vi "luch 2 in 1.vi"() -> ()   [LabVIEW 2016]
panel:
  out "Time Stamp":T1
  in  "stop":T2
  out "VISA resource name out":string
  out "I: DZ2K1W":string
  out "DZ2K1W":bool
  out "I: BZ2K1W":string
  out "BZ2K1W":bool
  out "I: BZ1K1W":string
  out "BZ1K1W":bool
  out "I: DZ1K1W":string
  out "DZ1K1W":bool
  out "I: F0-ethernet 5":string
  in  "F0-ethernet 5":bool
  out "F0-e 5":bool
  in  "GF":bool
  in  "FI":bool
  in  "F-R VISAR 4":bool
  in  "F-R VISAR 3":bool
  out "I: BZ1K2W":string
  out "BZ1K2W":bool
  out "I: DZ1K2W":string
  out "DZ1K2W":bool
  out "I: F0-ethernet 4":string
  in  "F0-ethernet 4":bool
  out "F0-e 4":bool
  out "I: BZ2K2W":string
  out "I: DZ2K2W":string
  out "DZ2K2W":bool
  out "BZ2K2W":bool
  in  "BK3":bool
  in  "BK 2":bool
  in  "BK1":bool
  in  "Kamera Y":bool
  out "mod 02":string
  out "mod 01":string
  in  "Setup":bool
  in  "Values start":T3=5 items=["External rising edge"=1, "Single shot internal rising edge"=3, "Single shot"=5]
  in  "DZ2K1W":bool
  in  "BZ2K1W":bool
  in  "BZ1K1W":bool
  in  "DZ1K1W":bool
  out "I F0-ethernet 1":string
  in  "F0-ethernet 1":bool
  out "F0-e 3":bool
  out "I: GF":string
  out "GF":bool
  in  "Delay D (0 s)":ext=100.0
  in  "GF":bool
  out "I: FI":string
  out "FI":bool
  in  "Delay C (0 s)":ext=100.0
  in  "FI":bool
  in  "F-R VISAR1":bool
  in  "Delay A (0 s)":ext=100.0
  out "F-R VISAR 1":bool
  out "I: F-R VISAR 1":string
  out "F-R VISAR 2":bool
  out "I: F-R VISAR 2":string
  in  "F-R VISAR2":bool
  in  "Delay B (0 s)":ext=100.0
  out "I F0-ethernet 3":string
  in  "F0-ethernet 3":bool
  out "F0-e 1":bool
  out "I: PZS 2 DOP":string
  out "I: PZS 1 DOP":string
  in  "PZS 2 DOP":bool
  in  "PZS 1 DOP":bool
  out "PZS 2 DOP":bool
  out "PZS 1 DOP":bool
  in  "BZ1K2W":bool
  in  "DZ1K2W":bool
  in  "BZ2K2W":bool
  in  "DZ2K2W":bool
  out "I: BK3":string
  out "BK3":bool
  in  "Delay H (0 s)":ext=100.0
  in  "BK3":bool
  in  "Delay G (0 s)":ext=100.0
  in  "BK2":bool
  out "I: BK2":string
  out "BK2":bool
  in  "Delay F (0 s)":ext=100.0
  in  "BK1":bool
  out "I: BK1":string
  out "BK1":bool
  out "I F0-ethernet 2":string
  in  "Delay E (0 s)":ext=100.0
  in  "Kamera Y":bool
  out "I: Kamera Y":string
  out "Kamera Y":bool
  in  "F0-ethernet 2":bool
  out "F0-e 2":bool
  out "error out 2":errorcluster
  out "I 0_3":string
  in  "rele 0_6":bool
  out "modul 03":string
  out "0_3":bool
  out "error out":errorcluster
  # "W1"
  # "Current(A)"
  # "FO-ETHERNET ¹5"
  # "2 CHANAL DZ"
  # "1 CHANAL DZ"
  # "Current(A)"
  # "Current(A)"
  # "2 CHANAL BZ"
  # "1 CHANAL BZ"
  # "Current(A)"
  # "Current(A)"
  # "W2"
  # "Current(A)"
  # "FO-ETHERNET ¹4"
  # "1 CHANAL DZ"
  # "2 CHANAL DZ"
  # "Current(A)"
  # "Current(A)"
  # "1 CHANAL BZ"
  # "2 CHANAL BZ"
  # "Current(A)"
  # "Current(A)"
  # "Current(A)"
  # "FO-ETHERNET ¹1"
  # "VISAR ¹2"
  # "VISAR ¹1"
  # "Current(A)"
  # "Current(A)"
  # "Delay (100~1099ns)"
  # "Delay (100~1099ns)"
  # "FORM IMPULSE"
  # "DEEP FRONT"
  # "Current(A)"
  # "Current(A)"
  # "Delay (100~1099ns)"
  # "Delay (100~1099ns)"
  # "Current(A)"
  # "FO-ETHERNET ¹3"
  # "PZS ¹1"
  # "PZS ¹2"
  # "Current(A)"
  # "Current(A)"
  # "Current(A)"
  # "FO-ETHERNET ¹2"
  # "KAMERA Y"
  # "KAMERA B1"
  # "Current(A)"
  # "Current(A)"
  # "Delay (100~1099ns)"
  # "Delay (100~1099ns)"
  # "KAMERA B2"
  # "KAMERA B3"
  # "Current(A)"
  # "Current(A)"
  # "Delay (100~1099ns)"
  # "Delay (100~1099ns)"
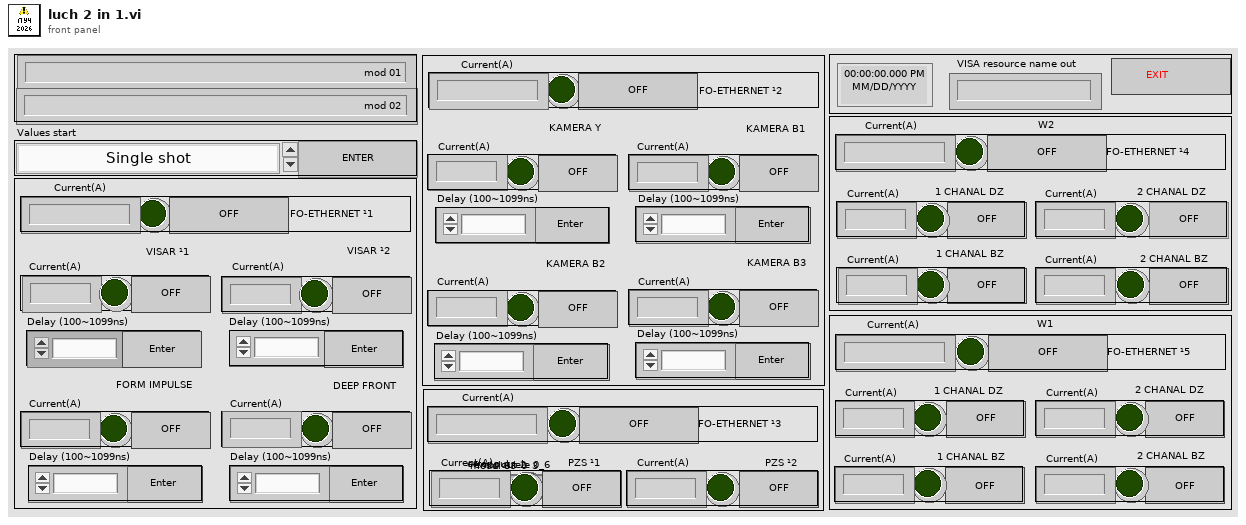
[diagram p1: front panel]
types:
  T1 = typedef "Control 4.ctl" = timestamp
  T2 = typedef "Control 1.ctl" = bool
  T3 = typedef "Control 2.ctl" = u16
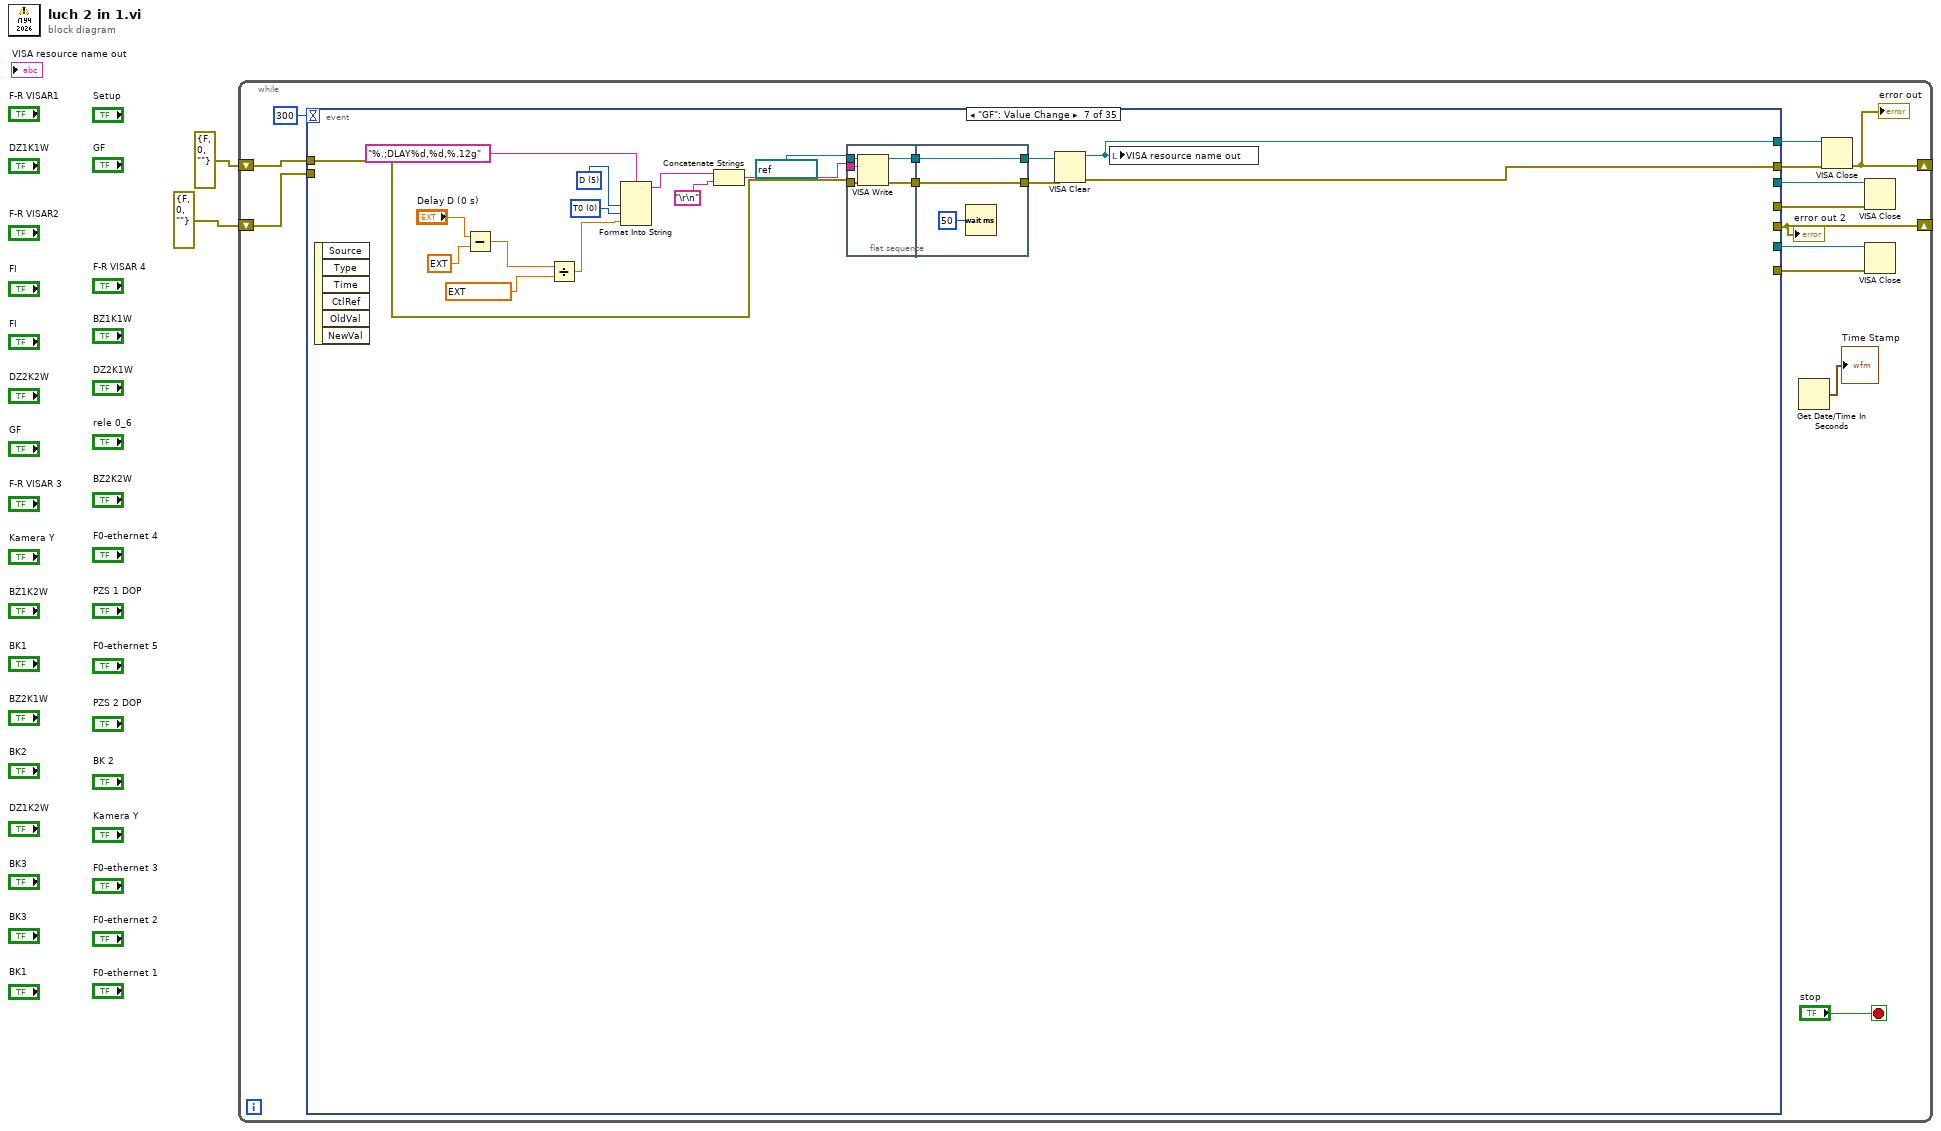
[diagram p0: block diagram]
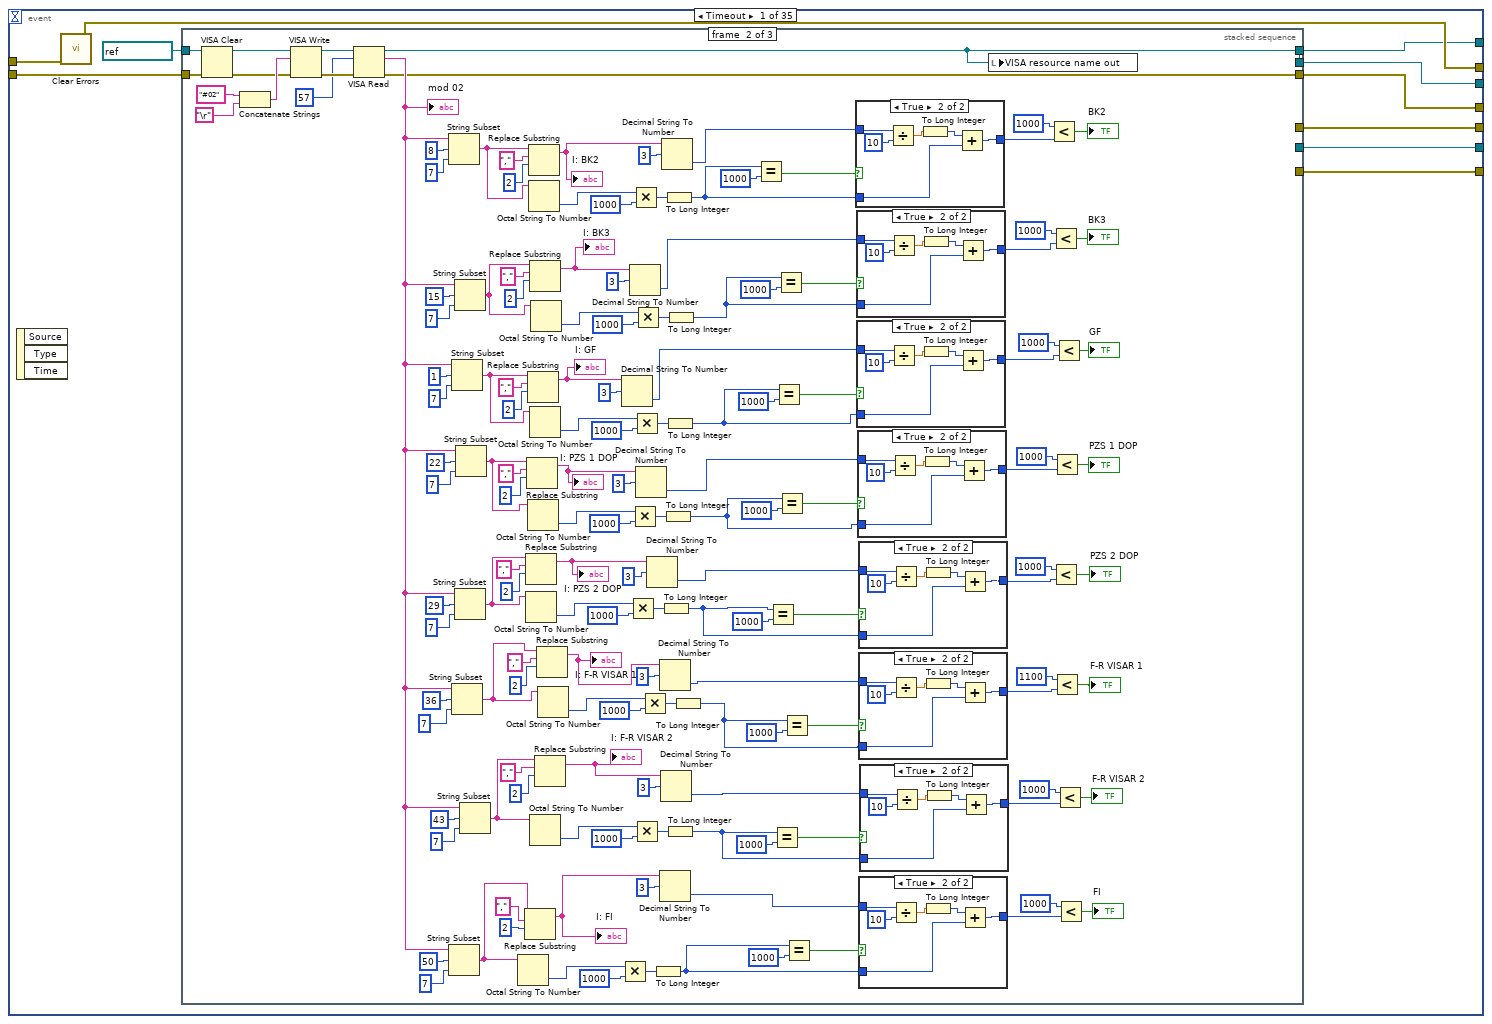
[diagram p2: hidden frame]
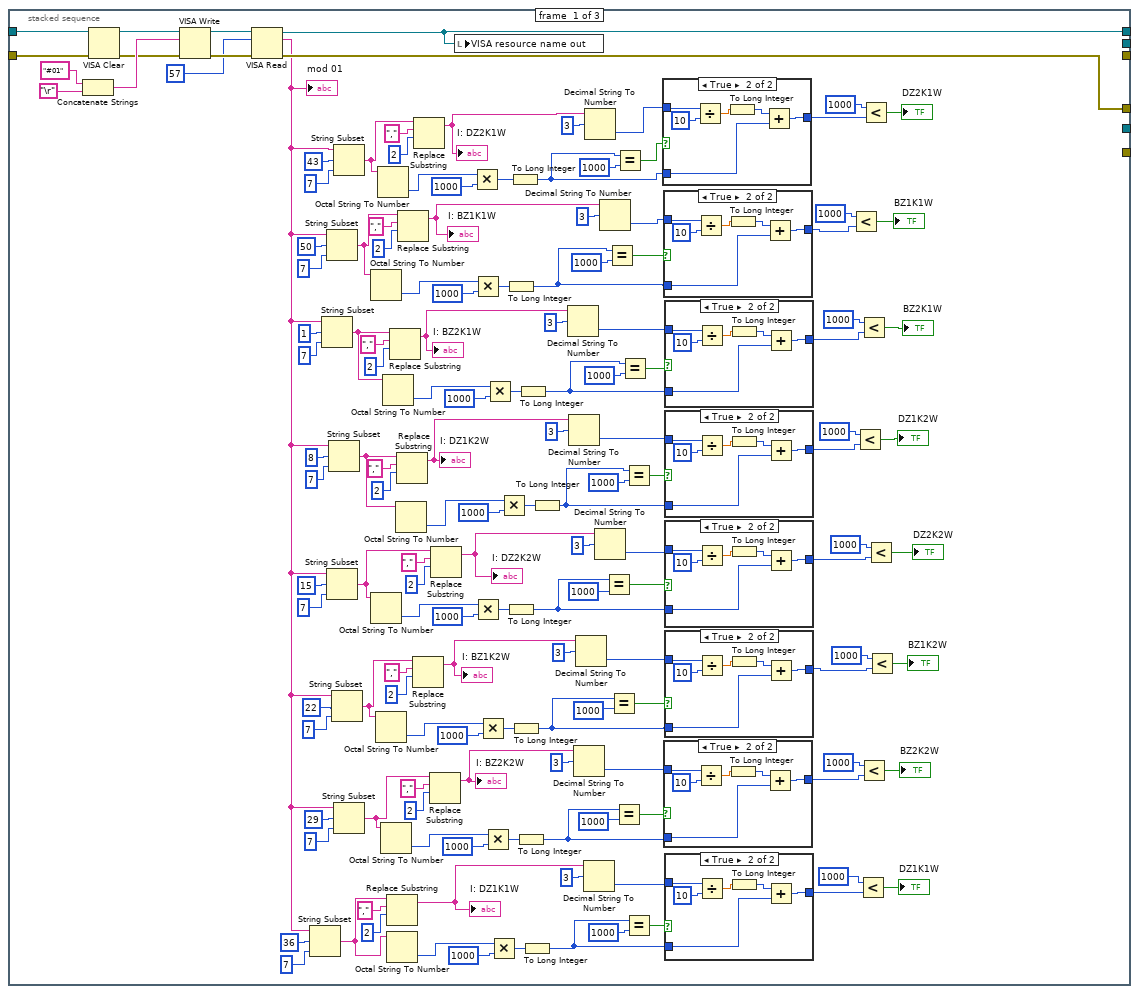
[diagram p3: hidden frame]
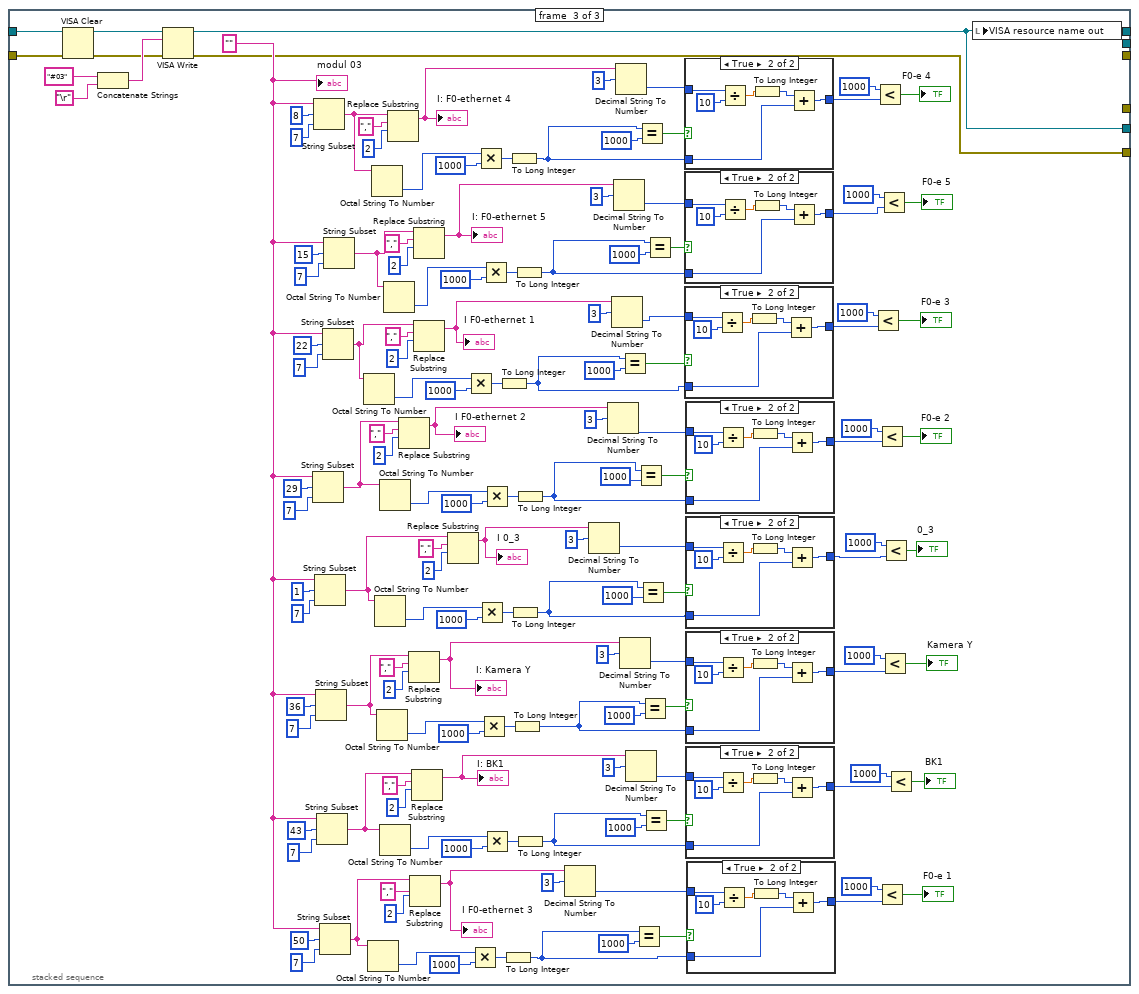
[diagram p20: hidden frame]
diagram:
  n1 = while {
    shift-right: [w13] -> _
    shift-left: errorcluster {"status"=FALSE, "code"=0, "source"=""} ("error out") -> [w15]
    shift-right: [w6] -> _
    shift-left: errorcluster {"status"=FALSE, "code"=0, "source"=""} ("error out") -> [w14]
    stop <- "stop" stop-if-true
    n2 = event shown="[6] \"GF\": Value Change" {
      selector: _ -> [_ _ _ _ _ _ _ _ _ _ _ _ _ _ _ _ _ _ _ _ _ _ _ _ _ _ _ _ _ _ _ _ _ _ _]
      dyn-events: _ -> [_ _ _ _ _ _ _ _ _ _ _ _ _ _ _ _ _ _ _ _ _ _ _ _ _ _ _ _ _ _ _ _ _ _ _]
      timeout: 300 -> [_ _ _ _ _ _ _ _ _ _ _ _ _ _ _ _ _ _ _ _ _ _ _ _ _ _ _ _ _ _ _ _ _ _ _]
      tunnel: [w24 w642 w645 w715 w742 w770 w796 w823 w849 w877 w904 _ _ _ _ _ _ _ _ _ _ _ _ _ _ _ _ _ _ _ _ _ _ _ _] -> w7
      tunnel: w15 -> [w25 w643 w647 w718 w745 w772 w799 w826 w853 w880 w907 _ _ _ _ _ _ _ _ _ _ _ _ _ _ _ _ _ _ _ _ _ _ _ _]
      tunnel: w14 -> [w22 w639 _ _ _ _ _ _ _ _ _ w929 w957 w990 w1021 w1052 w1083 w1114 w1145 w1176 w1208 w1238 w1269 w1300 w1331 w1362 w1394 w1424 w1455 w1486 w1517 w1548 w1579 w1610 w1641]
      tunnel: [w21 w638 _ _ _ _ _ _ _ _ _ w925 w956 w987 w1018 w1050 w1080 w1112 w1142 w1173 w1204 w1235 w1266 w1297 w1328 w1359 w1390 w1421 w1452 w1483 w1514 w1545 w1576 w1607 w1638] -> w6
      tunnel: [w20 _ w644 w711 w738 w765 w792 w819 w846 w873 w900 w922 w953 w984 w1015 w1046 w1077 w1108 w1139 w1170 w1201 w1232 w1263 w1294 w1325 w1356 w1387 w1418 w1449 w1480 w1511 w1542 w1573 w1604 w1635] -> w12
      tunnel: [w19 _ _ _ _ _ _ _ _ _ _ _ _ _ _ _ _ _ _ _ _ _ _ _ _ _ _ _ _ _ _ _ _ _ _] -> w11
      tunnel: [w18 _ _ _ _ _ _ _ _ _ _ _ _ _ _ _ _ _ _ _ _ _ _ _ _ _ _ _ _ _ _ _ _ _ _] -> w10
      tunnel: [w17 _ _ _ _ _ _ _ _ _ _ _ _ _ _ _ _ _ _ _ _ _ _ _ _ _ _ _ _ _ _ _ _ _ _] -> w9
      tunnel: [w16 _ _ _ _ _ _ _ _ _ _ _ _ _ _ _ _ _ _ _ _ _ _ _ _ _ _ _ _ _ _ _ _ _ _] -> w8
      event Timeout {
        n3 = event-data() -> ()  [unwired: 1 in, 3 out]
        n4 = call <vilib>:"Clear Errors.vi"("error in (no error)"=w25) -> ("error out"=w24:errorcluster)  [unwired: 5 in, 1 out]
        n5 = stacked-sequence {
          tunnel: refnum<visa-resource-name> "Adam" ("VISA resource name") -> [w102 w306 w530]
          tunnel: [w136 _ _] -> w21
          tunnel: w22 -> [w101 w308 w527]
          tunnel: [w98 _ _] -> w20
          tunnel: [_ w304 _] -> w19
          tunnel: [_ w303 _] -> w18
          tunnel: [_ _ w510] -> w17
          tunnel: [_ _ w509] -> w16
          frame #0 {
            n6 = Concatenate Strings("#01" ("string"), "\r") -> (w174:string)
            n7 = VISA Clear(VISA resource name=w102, error in (no error)=w101) -> (VISA resource name out=w99:refnum<visa-resource-name>, error out=w100:errorcluster)
            n8 = VISA Write(VISA resource name=w99, write buffer=w174, error in (no error)=w100) -> (VISA resource name out=w139:refnum<visa-resource-name>, error out=w138:errorcluster)  [unwired: 1 out]
            n9 = VISA Read(VISA resource name=w139, byte count=u32 57, error in (no error)=w138) -> (VISA resource name out=w98:refnum<visa-resource-name>, read buffer=w119:string, error out=w136:errorcluster)  [unwired: 1 out]
            "mod 01" <- w119
            n10 = String Subset(string=w119, offset (0)=36, length (rest)=7 ("length (rest)")) -> (substring=w93:string)
            n11 = String Subset(string=w119, offset (0)=1, length (rest)=7 ("length (rest)")) -> (substring=w48:string)
            n12 = String Subset(string=w119, offset (0)=50, length (rest)=7 ("length (rest)")) -> (substring=w38:string)
            n13 = String Subset(string=w119, offset (0)=15, length (rest)=7 ("length (rest)")) -> (substring=w66:string)
            n14 = String Subset(string=w119, offset (0)=8, length (rest)=7 ("length (rest)")) -> (substring=w53:string)
            n15 = String Subset(string=w119, offset (0)=22, length (rest)=7 ("length (rest)")) -> (substring=w71:string)
            n16 = String Subset(string=w119, offset (0)=43, length (rest)=7 ("length (rest)")) -> (substring=w29:string)
            n17 = String Subset(string=w119, offset (0)=29, length (rest)=7 ("length (rest)")) -> (substring=w83:string)
            n18 = Octal String To Number(4:w38) -> (0:w42:u32)  [unwired: 2 in, 1 out]
            n19 = Octal String To Number(4:w66) -> (0:w70:u32)  [unwired: 2 in, 1 out]
            n20 = Octal String To Number(4:w71) -> (0:w77:u32)  [unwired: 2 in, 1 out]
            n21 = Octal String To Number(4:w29) -> (0:w33:u32)  [unwired: 2 in, 1 out]
            n22 = Octal String To Number(4:w83) -> (0:w86:u32)  [unwired: 2 in, 1 out]
            n23 = Octal String To Number(4:w48) -> (0:w52:u32)  [unwired: 2 in, 1 out]
            n24 = Replace Substring(3:2 ("offset (0)"), 4:"," ("substring (\"\")"), 5:w93) -> (1:w107:string)  [unwired: 1 in, 1 out]
            "I: DZ1K1W" <- w107
            n25 = Octal String To Number(4:w93) -> (0:w97:u32)  [unwired: 2 in, 1 out]
            n26 = Replace Substring(3:2 ("offset (0)"), 4:"," ("substring (\"\")"), 5:w48) -> (1:w118:string)  [unwired: 1 in, 1 out]
            "I: BZ2K1W" <- w118
            n27 = Octal String To Number(4:w53) -> (0:w61:u32)  [unwired: 2 in, 1 out]
            n28 = Replace Substring(3:2 ("offset (0)"), 4:"," ("substring (\"\")"), 5:w53) -> (1:w116:string)  [unwired: 1 in, 1 out]
            "I: DZ1K2W" <- w116
            n29 = Replace Substring(3:2 ("offset (0)"), 4:"," ("substring (\"\")"), 5:w38) -> (1:w104:string)  [unwired: 1 in, 1 out]
            "I: BZ1K1W" <- w104
            n30 = Replace Substring(3:2 ("offset (0)"), 4:"," ("substring (\"\")"), 5:w71) -> (1:w112:string)  [unwired: 1 in, 1 out]
            "I: BZ1K2W" <- w112
            n31 = Replace Substring(3:2 ("offset (0)"), 4:"," ("substring (\"\")"), 5:w29) -> (1:w105:string)  [unwired: 1 in, 1 out]
            "I: DZ2K1W" <- w105
            n32 = Replace Substring(3:2 ("offset (0)"), 4:"," ("substring (\"\")"), 5:w83) -> (1:w110:string)  [unwired: 1 in, 1 out]
            "I: BZ2K2W" <- w110
            n33 = Replace Substring(3:2 ("offset (0)"), 4:"," ("substring (\"\")"), 5:w66) -> (1:w114:string)  [unwired: 1 in, 1 out]
            "I: DZ2K2W" <- w114
            n34 = local write "VISA resource name out"(w98) -> ()
            n35 = Multiply(x=w33, y=u32 1000) -> (x*y=w31:u32)
            n36 = Multiply(x=w42, y=u32 1000) -> (x*y=w40:u32)
            n37 = Multiply(x=w70, y=u32 1000) -> (x*y=w68:u32)
            n38 = Multiply(x=w77, y=u32 1000) -> (x*y=w75:u32)
            n39 = Multiply(x=w86, y=u32 1000) -> (x*y=w84:u32)
            n40 = Multiply(x=w52, y=u32 1000) -> (x*y=w50:u32)
            n41 = Multiply(x=w97, y=u32 1000) -> (x*y=w95:u32)
            n42 = Multiply(x=w61, y=u32 1000) -> (x*y=w59:u32)
            n43 = To Long Integer(number=w40) -> (32bit integer=w37:i32)
            n44 = To Long Integer(number=w68) -> (32bit integer=w65:i32)
            n45 = To Long Integer(number=w31) -> (32bit integer=w28:i32)
            n46 = To Long Integer(number=w75) -> (32bit integer=w73:i32)
            n47 = To Long Integer(number=w84) -> (32bit integer=w80:i32)
            n48 = To Long Integer(number=w50) -> (32bit integer=w47:i32)
            n49 = To Long Integer(number=w95) -> (32bit integer=w91:i32)
            n50 = To Long Integer(number=w59) -> (32bit integer=w56:i32)
            n51 = Decimal String To Number(string=w118, offset=3) -> (number=w44:i32)  [unwired: 1 in, 1 out]
            n52 = Decimal String To Number(string=w116, offset=3) -> (number=w54:i32)  [unwired: 1 in, 1 out]
            n53 = Decimal String To Number(string=w110, offset=3) -> (number=w87:i32)  [unwired: 1 in, 1 out]
            n54 = Decimal String To Number(string=w112, offset=3) -> (number=w78:i32)  [unwired: 1 in, 1 out]
            n55 = Decimal String To Number(string=w107, offset=3) -> (number=w90:i32)  [unwired: 1 in, 1 out]
            n56 = Decimal String To Number(string=w105, offset=3) -> (number=w26:i32)  [unwired: 1 in, 1 out]
            n57 = Decimal String To Number(string=w114, offset=3) -> (number=w62:i32)  [unwired: 1 in, 1 out]
            n58 = Decimal String To Number(string=w104, offset=3) -> (number=w35:i32)  [unwired: 1 in, 1 out]
            n59 = Equal?(x=w65, y=1000) -> (x = y?=w64:bool)
            n60 = Equal?(x=w37, y=1000) -> (x = y?=w36:bool)
            n61 = Equal?(x=w73, y=1000) -> (x = y?=w72:bool)
            n62 = Equal?(x=w80, y=1000) -> (x = y?=w81:bool)
            n63 = Equal?(x=w28, y=1000) -> (x = y?=w27:bool)
            n64 = Equal?(x=w47, y=1000) -> (x = y?=w46:bool)
            n65 = Equal?(x=w56, y=1000) -> (x = y?=w57:bool)
            n66 = Equal?(x=w91, y=1000) -> (x = y?=w92:bool)
            n67 = case shown="True" w27 {
              tunnel: w26 -> [w175 w181]
              tunnel: w28 -> [_ w179]
              tunnel: [w175 w178] -> w34
              frame False {
              }
              frame True {
                n68 = Divide(x=w181, y=10) -> (x/y=w177:dbl)
                n69 = To Long Integer(number=w177) -> (32bit integer=w176:i32)
                n70 = Add(x=w176, y=w179) -> (x+y=w178:i32)
              }
            }
            n71 = case shown="True" w36 {
              tunnel: w35 -> [w182 w188]
              tunnel: w37 -> [_ w186]
              tunnel: [w182 w185] -> w43
              frame False {
              }
              frame True {
                n72 = Divide(x=w188, y=10) -> (x/y=w184:dbl)
                n73 = To Long Integer(number=w184) -> (32bit integer=w183:i32)
                n74 = Add(x=w183, y=w186) -> (x+y=w185:i32)
              }
            }
            n75 = case shown="True" w81 {
              tunnel: w87 -> [w217 w223]
              tunnel: w80 -> [_ w221]
              tunnel: [w217 w220] -> w88
              frame False {
              }
              frame True {
                n76 = Divide(x=w223, y=10) -> (x/y=w219:dbl)
                n77 = To Long Integer(number=w219) -> (32bit integer=w218:i32)
                n78 = Add(x=w218, y=w221) -> (x+y=w220:i32)
              }
            }
            n79 = case shown="True" w46 {
              tunnel: w44 -> [w189 w195]
              tunnel: w47 -> [_ w193]
              tunnel: [w189 w192] -> w45
              frame False {
              }
              frame True {
                n80 = Divide(x=w195, y=10) -> (x/y=w191:dbl)
                n81 = To Long Integer(number=w191) -> (32bit integer=w190:i32)
                n82 = Add(x=w190, y=w193) -> (x+y=w192:i32)
              }
            }
            n83 = case shown="True" w57 {
              tunnel: w54 -> [w196 w202]
              tunnel: w56 -> [_ w200]
              tunnel: [w196 w199] -> w55
              frame False {
              }
              frame True {
                n84 = Divide(x=w202, y=10) -> (x/y=w198:dbl)
                n85 = To Long Integer(number=w198) -> (32bit integer=w197:i32)
                n86 = Add(x=w197, y=w200) -> (x+y=w199:i32)
              }
            }
            n87 = case shown="True" w64 {
              tunnel: w62 -> [w203 w209]
              tunnel: w65 -> [_ w207]
              tunnel: [w203 w206] -> w63
              frame False {
              }
              frame True {
                n88 = Divide(x=w209, y=10) -> (x/y=w205:dbl)
                n89 = To Long Integer(number=w205) -> (32bit integer=w204:i32)
                n90 = Add(x=w204, y=w207) -> (x+y=w206:i32)
              }
            }
            n91 = case shown="True" w72 {
              tunnel: w78 -> [w210 w216]
              tunnel: w73 -> [_ w214]
              tunnel: [w210 w213] -> w79
              frame False {
              }
              frame True {
                n92 = Divide(x=w216, y=10) -> (x/y=w212:dbl)
                n93 = To Long Integer(number=w212) -> (32bit integer=w211:i32)
                n94 = Add(x=w211, y=w214) -> (x+y=w213:i32)
              }
            }
            n95 = case shown="True" w92 {
              tunnel: w90 -> [w224 w230]
              tunnel: w91 -> [_ w228]
              tunnel: [w224 w227] -> w89
              frame False {
              }
              frame True {
                n96 = Divide(x=w230, y=10) -> (x/y=w226:dbl)
                n97 = To Long Integer(number=w226) -> (32bit integer=w225:i32)
                n98 = Add(x=w225, y=w228) -> (x+y=w227:i32)
              }
            }
            n99 = Less?(x=1000, y=w43) -> (x < y?=→"BZ1K1W":bool)
            n100 = Less?(x=1000, y=w55) -> (x < y?=→"DZ1K2W":bool)
            n101 = Less?(x=1000, y=w89) -> (x < y?=→"DZ1K1W":bool)
            n102 = Less?(x=1000, y=w45) -> (x < y?=→"BZ2K1W":bool)
            n103 = Less?(x=1000, y=w88) -> (x < y?=→"BZ2K2W":bool)
            n104 = Less?(x=1000, y=w34) -> (x < y?=→"DZ2K1W":bool)
            n105 = Less?(x=1000, y=w63) -> (x < y?=→"DZ2K2W":bool)
            n106 = Less?(x=1000, y=w79) -> (x < y?=→"BZ1K2W":bool)
          }
          frame #1 {
            n107 = VISA Clear(VISA resource name=w306, error in (no error)=w308) -> (VISA resource name out=w305:refnum<visa-resource-name>, error out=w307:errorcluster)
            n108 = Concatenate Strings("#02" ("string"), "\r") -> (w379:string)
            n109 = VISA Write(VISA resource name=w305, write buffer=w379, error in (no error)=w307) -> (VISA resource name out=w344:refnum<visa-resource-name>, error out=w343:errorcluster)  [unwired: 1 out]
            n110 = VISA Read(VISA resource name=w344, byte count=u32 57, error in (no error)=w343) -> (VISA resource name out=w304:refnum<visa-resource-name>, read buffer=w325:string, error out=w303:errorcluster)  [unwired: 1 out]
            "mod 02" <- w325
            n111 = String Subset(string=w325, offset (0)=8, length (rest)=7 ("length (rest)")) -> (substring=w235:string)
            n112 = String Subset(string=w325, offset (0)=50, length (rest)=7 ("length (rest)")) -> (substring=w302:string)
            n113 = String Subset(string=w325, offset (0)=1, length (rest)=7 ("length (rest)")) -> (substring=w253:string)
            n114 = String Subset(string=w325, offset (0)=36, length (rest)=7 ("length (rest)")) -> (substring=w280:string)
            n115 = String Subset(string=w325, offset (0)=15, length (rest)=7 ("length (rest)")) -> (substring=w241:string)
            n116 = String Subset(string=w325, offset (0)=29, length (rest)=7 ("length (rest)")) -> (substring=w272:string)
            n117 = String Subset(string=w325, offset (0)=22, length (rest)=7 ("length (rest)")) -> (substring=w262:string)
            n118 = String Subset(string=w325, offset (0)=43, length (rest)=7 ("length (rest)")) -> (substring=w289:string)
            n119 = Octal String To Number(4:w302) -> (0:w301:u32)  [unwired: 2 in, 1 out]
            n120 = Replace Substring(3:2 ("offset (0)"), 4:"," ("substring (\"\")"), 5:w302) -> (1:w311:string)  [unwired: 1 in, 1 out]
            "I: FI" <- w311
            n121 = Replace Substring(3:2 ("offset (0)"), 4:"," ("substring (\"\")"), 5:w272) -> (1:w315:string)  [unwired: 1 in, 1 out]
            "I: PZS 2 DOP" <- w315
            n122 = Octal String To Number(4:w272) -> (0:w276:u32)  [unwired: 2 in, 1 out]
            n123 = Replace Substring(3:2 ("offset (0)"), 4:"," ("substring (\"\")"), 5:w262) -> (1:w318:string)  [unwired: 1 in, 1 out]
            "I: PZS 1 DOP" <- w318
            n124 = Replace Substring(3:2 ("offset (0)"), 4:"," ("substring (\"\")"), 5:w253) -> (1:w323:string)  [unwired: 1 in, 1 out]
            "I: GF" <- w323
            n125 = Octal String To Number(4:w262) -> (0:w266:u32)  [unwired: 2 in, 1 out]
            n126 = Replace Substring(3:2 ("offset (0)"), 4:"," ("substring (\"\")"), 5:w235) -> (1:w321:string)  [unwired: 1 in, 1 out]
            "I: BK2" <- w321
            n127 = Octal String To Number(4:w235) -> (0:w239:u32)  [unwired: 2 in, 1 out]
            n128 = Replace Substring(3:2 ("offset (0)"), 4:"," ("substring (\"\")"), 5:w241) -> (1:w320:string)  [unwired: 1 in, 1 out]
            "I: BK3" <- w320
            n129 = Octal String To Number(4:w253) -> (0:w257:u32)  [unwired: 2 in, 1 out]
            n130 = Octal String To Number(4:w289) -> (0:w293:u32)  [unwired: 2 in, 1 out]
            n131 = Octal String To Number(4:w241) -> (0:w247:u32)  [unwired: 2 in, 1 out]
            n132 = Replace Substring(3:2 ("offset (0)"), 4:"," ("substring (\"\")"), 5:w289) -> (1:w312:string)  [unwired: 1 in, 1 out]
            "I: F-R VISAR 2" <- w312
            n133 = Replace Substring(3:2 ("offset (0)"), 4:"," ("substring (\"\")"), 5:w280) -> (1:w313:string)  [unwired: 1 in, 1 out]
            "I: F-R VISAR 1" <- w313
            n134 = Octal String To Number(4:w280) -> (0:w284:u32)  [unwired: 2 in, 1 out]
            n135 = Multiply(x=w301, y=u32 1000) -> (x*y=w299:u32)
            n136 = Decimal String To Number(string=w323, offset=3) -> (number=w250:i32)  [unwired: 1 in, 1 out]
            n137 = Multiply(x=w276, y=u32 1000) -> (x*y=w274:u32)
            n138 = Decimal String To Number(string=w320, offset=3) -> (number=w240:i32)  [unwired: 1 in, 1 out]
            n139 = Multiply(x=w266, y=u32 1000) -> (x*y=w264:u32)
            n140 = Multiply(x=w239, y=u32 1000) -> (x*y=w237:u32)
            n141 = Multiply(x=w257, y=u32 1000) -> (x*y=w255:u32)
            n142 = Multiply(x=w293, y=u32 1000) -> (x*y=w291:u32)
            n143 = Multiply(x=w247, y=u32 1000) -> (x*y=w245:u32)
            n144 = Decimal String To Number(string=w318, offset=3) -> (number=w258:i32)  [unwired: 1 in, 1 out]
            n145 = Multiply(x=w284, y=u32 1000) -> (x*y=w282:u32)
            n146 = Decimal String To Number(string=w315, offset=3) -> (number=w270:i32)  [unwired: 1 in, 1 out]
            n147 = To Long Integer(number=w299) -> (32bit integer=w295:i32)
            n148 = Decimal String To Number(string=w313, offset=3) -> (number=w277:i32)  [unwired: 1 in, 1 out]
            n149 = Decimal String To Number(string=w311, offset=3) -> (number=w296:i32)  [unwired: 1 in, 1 out]
            n150 = To Long Integer(number=w274) -> (32bit integer=w267:i32)
            n151 = Decimal String To Number(string=w312, offset=3) -> (number=w286:i32)  [unwired: 1 in, 1 out]
            n152 = Decimal String To Number(string=w321, offset=3) -> (number=w231:i32)  [unwired: 1 in, 1 out]
            n153 = To Long Integer(number=w264) -> (32bit integer=w259:i32)
            n154 = To Long Integer(number=w237) -> (32bit integer=w232:i32)
            n155 = To Long Integer(number=w255) -> (32bit integer=w251:i32)
            n156 = To Long Integer(number=w291) -> (32bit integer=w287:i32)
            n157 = To Long Integer(number=w245) -> (32bit integer=w242:i32)
            n158 = To Long Integer(number=w282) -> (32bit integer=w278:i32)
            n159 = Equal?(x=w232, y=1000) -> (x = y?=w233:bool)
            n160 = Equal?(x=w267, y=1000) -> (x = y?=w271:bool)
            n161 = Equal?(x=w287, y=1000) -> (x = y?=w288:bool)
            n162 = Equal?(x=w251, y=1000) -> (x = y?=w252:bool)
            n163 = Equal?(x=w242, y=1000) -> (x = y?=w243:bool)
            n164 = Equal?(x=w259, y=1000) -> (x = y?=w260:bool)
            n165 = Equal?(x=w278, y=1000) -> (x = y?=w279:bool)
            n166 = Equal?(x=w295, y=1000) -> (x = y?=w297:bool)
            n167 = case shown="True" w233 {
              tunnel: w231 -> [w380 w386]
              tunnel: w232 -> [_ w384]
              tunnel: [w380 w383] -> w234
              frame False {
              }
              frame True {
                n168 = Divide(x=w386, y=10) -> (x/y=w382:dbl)
                n169 = To Long Integer(number=w382) -> (32bit integer=w381:i32)
                n170 = Add(x=w381, y=w384) -> (x+y=w383:i32)
              }
            }
            n171 = case shown="True" w243 {
              tunnel: w240 -> [w387 w393]
              tunnel: w242 -> [_ w391]
              tunnel: [w387 w390] -> w248
              frame False {
              }
              frame True {
                n172 = Divide(x=w393, y=10) -> (x/y=w389:dbl)
                n173 = To Long Integer(number=w389) -> (32bit integer=w388:i32)
                n174 = Add(x=w388, y=w391) -> (x+y=w390:i32)
              }
            }
            n175 = case shown="True" w252 {
              tunnel: w250 -> [w394 w400]
              tunnel: w251 -> [_ w398]
              tunnel: [w394 w397] -> w249
              frame False {
              }
              frame True {
                n176 = Divide(x=w400, y=10) -> (x/y=w396:dbl)
                n177 = To Long Integer(number=w396) -> (32bit integer=w395:i32)
                n178 = Add(x=w395, y=w398) -> (x+y=w397:i32)
              }
            }
            n179 = case shown="True" w260 {
              tunnel: w258 -> [w401 w407]
              tunnel: w259 -> [_ w405]
              tunnel: [w401 w404] -> w261
              frame False {
              }
              frame True {
                n180 = Divide(x=w407, y=10) -> (x/y=w403:dbl)
                n181 = To Long Integer(number=w403) -> (32bit integer=w402:i32)
                n182 = Add(x=w402, y=w405) -> (x+y=w404:i32)
              }
            }
            n183 = case shown="True" w271 {
              tunnel: w270 -> [w408 w414]
              tunnel: w267 -> [_ w412]
              tunnel: [w408 w411] -> w268
              frame False {
              }
              frame True {
                n184 = Divide(x=w414, y=10) -> (x/y=w410:dbl)
                n185 = To Long Integer(number=w410) -> (32bit integer=w409:i32)
                n186 = Add(x=w409, y=w412) -> (x+y=w411:i32)
              }
            }
            n187 = case shown="True" w279 {
              tunnel: w277 -> [w415 w421]
              tunnel: w278 -> [_ w419]
              tunnel: [w415 w418] -> w269
              frame False {
              }
              frame True {
                n188 = Divide(x=w421, y=10) -> (x/y=w417:dbl)
                n189 = To Long Integer(number=w417) -> (32bit integer=w416:i32)
                n190 = Add(x=w416, y=w419) -> (x+y=w418:i32)
              }
            }
            n191 = case shown="True" w297 {
              tunnel: w296 -> [w429 w435]
              tunnel: w295 -> [_ w433]
              tunnel: [w429 w432] -> w294
              frame False {
              }
              frame True {
                n192 = Divide(x=w435, y=10) -> (x/y=w431:dbl)
                n193 = To Long Integer(number=w431) -> (32bit integer=w430:i32)
                n194 = Add(x=w430, y=w433) -> (x+y=w432:i32)
              }
            }
            n195 = case shown="True" w288 {
              tunnel: w286 -> [w422 w428]
              tunnel: w287 -> [_ w426]
              tunnel: [w422 w425] -> w285
              frame False {
              }
              frame True {
                n196 = Divide(x=w428, y=10) -> (x/y=w424:dbl)
                n197 = To Long Integer(number=w424) -> (32bit integer=w423:i32)
                n198 = Add(x=w423, y=w426) -> (x+y=w425:i32)
              }
            }
            n199 = local write "VISA resource name out"(w304) -> ()
            n200 = Less?(x=1000, y=w234) -> (x < y?=→"BK2":bool)
            n201 = Less?(x=1000, y=w248) -> (x < y?=→"BK3":bool)
            n202 = Less?(x=1000, y=w268) -> (x < y?=→"PZS 2 DOP":bool)
            n203 = Less?(x=1000, y=w261) -> (x < y?=→"PZS 1 DOP":bool)
            n204 = Less?(x=1100, y=w269) -> (x < y?=→"F-R VISAR 1":bool)
            n205 = Less?(x=1000, y=w249) -> (x < y?=→"GF":bool)
            n206 = Less?(x=1000, y=w285) -> (x < y?=→"F-R VISAR 2":bool)
            n207 = Less?(x=1000, y=w294) -> (x < y?=→"FI":bool)
          }
          frame #2 {
            w526 = "" ("string")
            n208 = VISA Clear(VISA resource name=w530, error in (no error)=w527) -> (VISA resource name out=w528:refnum<visa-resource-name>, error out=w529:errorcluster)
            n209 = Concatenate Strings("#03" ("string"), "\r") -> (w581:string)
            n210 = VISA Write(VISA resource name=w528, write buffer=w581, error in (no error)=w529) -> (VISA resource name out=w509:refnum<visa-resource-name>, error out=w510:errorcluster)  [unwired: 1 out]
            n211 = String Subset(string=w526, offset (0)=29, length (rest)=7 ("length (rest)")) -> (substring=w465:string)
            n212 = String Subset(string=w526, offset (0)=8, length (rest)=7 ("length (rest)")) -> (substring=w438:string)
            n213 = String Subset(string=w526, offset (0)=1, length (rest)=7 ("length (rest)")) -> (substring=w476:string)
            n214 = String Subset(string=w526, offset (0)=36, length (rest)=7 ("length (rest)")) -> (substring=w482:string)
            n215 = String Subset(string=w526, offset (0)=43, length (rest)=7 ("length (rest)")) -> (substring=w492:string)
            n216 = String Subset(string=w526, offset (0)=50, length (rest)=7 ("length (rest)")) -> (substring=w499:string)
            n217 = String Subset(string=w526, offset (0)=22, length (rest)=7 ("length (rest)")) -> (substring=w456:string)
            n218 = String Subset(string=w526, offset (0)=15, length (rest)=7 ("length (rest)")) -> (substring=w449:string)
            n219 = Octal String To Number(4:w456) -> (0:w457:u32)  [unwired: 2 in, 1 out]
            n220 = Octal String To Number(4:w499) -> (0:w505:u32)  [unwired: 2 in, 1 out]
            n221 = Octal String To Number(4:w438) -> (0:w442:u32)  [unwired: 2 in, 1 out]
            n222 = Octal String To Number(4:w476) -> (0:w480:u32)  [unwired: 2 in, 1 out]
            n223 = Octal String To Number(4:w482) -> (0:w488:u32)  [unwired: 2 in, 1 out]
            n224 = Octal String To Number(4:w465) -> (0:w466:u32)  [unwired: 2 in, 1 out]
            n225 = Octal String To Number(4:w492) -> (0:w496:u32)  [unwired: 2 in, 1 out]
            n226 = Octal String To Number(4:w449) -> (0:w453:u32)  [unwired: 2 in, 1 out]
            n227 = Replace Substring(3:2 ("offset (0)"), 4:"," ("substring (\"\")"), 5:w438) -> (1:w523:string)  [unwired: 1 in, 1 out]
            "I: F0-ethernet 4" <- w523
            n228 = Replace Substring(3:2 ("offset (0)"), 4:"," ("substring (\"\")"), 5:w465) -> (1:w516:string)  [unwired: 1 in, 1 out]
            "I F0-ethernet 2" <- w516
            n229 = Replace Substring(3:2 ("offset (0)"), 4:"," ("substring (\"\")"), 5:w482) -> (1:w514:string)  [unwired: 1 in, 1 out]
            "I: Kamera Y" <- w514
            n230 = Replace Substring(3:2 ("offset (0)"), 4:"," ("substring (\"\")"), 5:w499) -> (1:w511:string)  [unwired: 1 in, 1 out]
            "I F0-ethernet 3" <- w511
            n231 = Replace Substring(3:2 ("offset (0)"), 4:"," ("substring (\"\")"), 5:w492) -> (1:w513:string)  [unwired: 1 in, 1 out]
            "I: BK1" <- w513
            n232 = Replace Substring(3:2 ("offset (0)"), 4:"," ("substring (\"\")"), 5:w449) -> (1:w521:string)  [unwired: 1 in, 1 out]
            "I: F0-ethernet 5" <- w521
            n233 = Replace Substring(3:2 ("offset (0)"), 4:"," ("substring (\"\")"), 5:w456) -> (1:w519:string)  [unwired: 1 in, 1 out]
            "I F0-ethernet 1" <- w519
            n234 = Replace Substring(3:2 ("offset (0)"), 4:"," ("substring (\"\")"), 5:w476) -> (1:w525:string)  [unwired: 1 in, 1 out]
            "I 0_3" <- w525
            n235 = Multiply(x=w457, y=u32 1000) -> (x*y=w459:u32)
            n236 = Multiply(x=w505, y=u32 1000) -> (x*y=w503:u32)
            n237 = Multiply(x=w442, y=u32 1000) -> (x*y=w440:u32)
            n238 = Multiply(x=w480, y=u32 1000) -> (x*y=w478:u32)
            n239 = Multiply(x=w488, y=u32 1000) -> (x*y=w486:u32)
            n240 = Multiply(x=w453, y=u32 1000) -> (x*y=w451:u32)
            n241 = Multiply(x=w466, y=u32 1000) -> (x*y=w468:u32)
            n242 = Multiply(x=w496, y=u32 1000) -> (x*y=w494:u32)
            n243 = To Long Integer(number=w459) -> (32bit integer=w455:i32)
            n244 = To Long Integer(number=w503) -> (32bit integer=w501:i32)
            n245 = To Long Integer(number=w440) -> (32bit integer=w437:i32)
            n246 = To Long Integer(number=w478) -> (32bit integer=w474:i32)
            n247 = To Long Integer(number=w486) -> (32bit integer=w484:i32)
            n248 = To Long Integer(number=w451) -> (32bit integer=w448:i32)
            n249 = To Long Integer(number=w468) -> (32bit integer=w464:i32)
            n250 = To Long Integer(number=w494) -> (32bit integer=w491:i32)
            n251 = Decimal String To Number(string=w511, offset=3) -> (number=w506:i32)  [unwired: 1 in, 1 out]
            n252 = Decimal String To Number(string=w525, offset=3) -> (number=w472:i32)  [unwired: 1 in, 1 out]
            n253 = Decimal String To Number(string=w516, offset=3) -> (number=w470:i32)  [unwired: 1 in, 1 out]
            n254 = Decimal String To Number(string=w519, offset=3) -> (number=w461:i32)  [unwired: 1 in, 1 out]
            n255 = Decimal String To Number(string=w521, offset=3) -> (number=w445:i32)  [unwired: 1 in, 1 out]
            n256 = Decimal String To Number(string=w523, offset=3) -> (number=w443:i32)  [unwired: 1 in, 1 out]
            n257 = Equal?(x=w455, y=1000) -> (x = y?=w454:bool)
            n258 = Decimal String To Number(string=w514, offset=3) -> (number=w481:i32)  [unwired: 1 in, 1 out]
            n259 = Decimal String To Number(string=w513, offset=3) -> (number=w497:i32)  [unwired: 1 in, 1 out]
            n260 = Equal?(x=w501, y=1000) -> (x = y?=w500:bool)
            n261 = Equal?(x=w464, y=1000) -> (x = y?=w463:bool)
            n262 = Equal?(x=w437, y=1000) -> (x = y?=w436:bool)
            n263 = Equal?(x=w474, y=1000) -> (x = y?=w475:bool)
            n264 = Equal?(x=w484, y=1000) -> (x = y?=w483:bool)
            n265 = Equal?(x=w491, y=1000) -> (x = y?=w490:bool)
            n266 = Equal?(x=w448, y=1000) -> (x = y?=w447:bool)
            n267 = case shown="True" w436 {
              tunnel: w443 -> [w582 w588]
              tunnel: w437 -> [_ w586]
              tunnel: [w582 w585] -> w444
              frame False {
              }
              frame True {
                n268 = Divide(x=w588, y=10) -> (x/y=w584:dbl)
                n269 = To Long Integer(number=w584) -> (32bit integer=w583:i32)
                n270 = Add(x=w583, y=w586) -> (x+y=w585:i32)
              }
            }
            n271 = case shown="True" w447 {
              tunnel: w445 -> [w589 w595]
              tunnel: w448 -> [_ w593]
              tunnel: [w589 w592] -> w446
              frame False {
              }
              frame True {
                n272 = Divide(x=w595, y=10) -> (x/y=w591:dbl)
                n273 = To Long Integer(number=w591) -> (32bit integer=w590:i32)
                n274 = Add(x=w590, y=w593) -> (x+y=w592:i32)
              }
            }
            n275 = case shown="True" w454 {
              tunnel: w461 -> [w596 w602]
              tunnel: w455 -> [_ w600]
              tunnel: [w596 w599] -> w462
              frame False {
              }
              frame True {
                n276 = Divide(x=w602, y=10) -> (x/y=w598:dbl)
                n277 = To Long Integer(number=w598) -> (32bit integer=w597:i32)
                n278 = Add(x=w597, y=w600) -> (x+y=w599:i32)
              }
            }
            n279 = case shown="True" w463 {
              tunnel: w470 -> [w603 w609]
              tunnel: w464 -> [_ w607]
              tunnel: [w603 w606] -> w471
              frame False {
              }
              frame True {
                n280 = Divide(x=w609, y=10) -> (x/y=w605:dbl)
                n281 = To Long Integer(number=w605) -> (32bit integer=w604:i32)
                n282 = Add(x=w604, y=w607) -> (x+y=w606:i32)
              }
            }
            n283 = case shown="True" w475 {
              tunnel: w472 -> [w610 w616]
              tunnel: w474 -> [_ w614]
              tunnel: [w610 w613] -> w473
              frame False {
              }
              frame True {
                n284 = Divide(x=w616, y=10) -> (x/y=w612:dbl)
                n285 = To Long Integer(number=w612) -> (32bit integer=w611:i32)
                n286 = Add(x=w611, y=w614) -> (x+y=w613:i32)
              }
            }
            n287 = case shown="True" w483 {
              tunnel: w481 -> [w617 w623]
              tunnel: w484 -> [_ w621]
              tunnel: [w617 w620] -> w489
              frame False {
              }
              frame True {
                n288 = Divide(x=w623, y=10) -> (x/y=w619:dbl)
                n289 = To Long Integer(number=w619) -> (32bit integer=w618:i32)
                n290 = Add(x=w618, y=w621) -> (x+y=w620:i32)
              }
            }
            n291 = case shown="True" w490 {
              tunnel: w497 -> [w624 w630]
              tunnel: w491 -> [_ w628]
              tunnel: [w624 w627] -> w498
              frame False {
              }
              frame True {
                n292 = Divide(x=w630, y=10) -> (x/y=w626:dbl)
                n293 = To Long Integer(number=w626) -> (32bit integer=w625:i32)
                n294 = Add(x=w625, y=w628) -> (x+y=w627:i32)
              }
            }
            n295 = case shown="True" w500 {
              tunnel: w506 -> [w631 w637]
              tunnel: w501 -> [_ w635]
              tunnel: [w631 w634] -> w507
              frame False {
              }
              frame True {
                n296 = Divide(x=w637, y=10) -> (x/y=w633:dbl)
                n297 = To Long Integer(number=w633) -> (32bit integer=w632:i32)
                n298 = Add(x=w632, y=w635) -> (x+y=w634:i32)
              }
            }
            n299 = Less?(x=1000, y=w462) -> (x < y?=→"F0-e 3":bool)
            n300 = Less?(x=1000, y=w444) -> (x < y?=→"F0-e 4":bool)
            n301 = Less?(x=1000, y=w471) -> (x < y?=→"F0-e 2":bool)
            n302 = Less?(x=1000, y=w507) -> (x < y?=→"F0-e 1":bool)
            n303 = Less?(x=1000, y=w446) -> (x < y?=→"F0-e 5":bool)
            n304 = Less?(x=1000, y=w489) -> (x < y?=→"Kamera Y":bool)
            n305 = Less?(x=1000, y=w473) -> (x < y?=→"0_3":bool)
            n306 = Less?(x=1000, y=w498) -> (x < y?=→"BK1":bool)
            n307 = local write "VISA resource name out"(w509) -> ()
            "modul 03" <- w526
          }
        }
      }
      event Value Change {
        n308 = event-data() -> ()  [unwired: 1 in, 6 out]
        n309 = VISA Close(VISA resource name=refnum<visa-resource-name> "DG645", error in (no error)=w643) -> (error out=w642:errorcluster)
        n310 = VISA Close(VISA resource name=refnum<visa-resource-name> "Adam", error in (no error)=w639) -> (error out=w638:errorcluster)
      }
      event "Setup": Value Change {
        n311 = event-data() -> ()  [unwired: 1 in, 6 out]
        n312 = Equal?(x="Values start", y=u16 5) -> (x = y?=w650:bool)
        n313 = Equal?(x="Values start", y=u16 3) -> (x = y?=w649:bool)
        n314 = Format Into String(format string="TSRC%d", "Values start") -> (resulting string=w646:string)  [unwired: 2 in, 1 out]
        n315 = Or(x=w649, y=w650) -> (x .or. y?=w648:bool)
        n316 = case shown="True" w648 {
          tunnel: w647 -> [w658 w684]
          tunnel: w646 -> [w657 w685]
          tunnel: [w656 w679] -> w645
          tunnel: [w655 w678] -> w644
          frame False {
            n317 = Concatenate Strings(w657, "\r\n") -> (w663:string)
            n318 = flat-sequence {
              tunnel: w663 -> [w670]
              tunnel: w658 -> [w669]
              tunnel: refnum<visa-resource-name> "DG645" ("VISA resource name") -> [w668]
              tunnel: [w667] -> w665
              tunnel: [w666] -> w664
              tunnel: [w672] -> w659
              tunnel: [w673] -> w660
              tunnel: w665 -> [w673]
              tunnel: w664 -> [w672]
              frame #0 {
                n319 = VISA Write(VISA resource name=w668, write buffer=w670, error in (no error)=w669) -> (VISA resource name out=w666:refnum<visa-resource-name>, error out=w667:errorcluster)  [unwired: 1 out]
              }
              frame #1 {
                n320 = Wait (ms)(milliseconds to wait=u32 50) -> ()  [unwired: 1 out]
              }
            }
            n321 = VISA Clear(VISA resource name=w659, error in (no error)=w660) -> (VISA resource name out=w655:refnum<visa-resource-name>, error out=w656:errorcluster)
          }
          frame True {
            n322 = Concatenate Strings(w685, "\r\n") -> (w688:string)
            n323 = flat-sequence {
              tunnel: w688 -> [w693]
              tunnel: w684 -> [w692]
              tunnel: refnum<visa-resource-name> "DG645" ("VISA resource name") -> [w691]
              tunnel: [w690] -> w675
              tunnel: [w689] -> w674
              tunnel: [w694] -> w677
              tunnel: [w695] -> w676
              tunnel: w675 -> [w694]
              tunnel: w674 -> [w695]
              tunnel: w677 -> [w699]
              tunnel: w676 -> [w698]
              tunnel: [w697] -> w683
              tunnel: [w696] -> w681
              tunnel: [w704] -> w682
              tunnel: w683 -> [w704]
              tunnel: [w703] -> w680
              tunnel: w681 -> [w703]
              frame #0 {
                n324 = VISA Write(VISA resource name=w691, write buffer=w693, error in (no error)=w692) -> (VISA resource name out=w689:refnum<visa-resource-name>, error out=w690:errorcluster)  [unwired: 1 out]
              }
              frame #1 {
              }
              frame #2 {
                n325 = Concatenate Strings("*TRG" ("string"), "\r\n") -> (w700:string)
                n326 = VISA Write(VISA resource name=w698, write buffer=w700, error in (no error)=w699) -> (VISA resource name out=w696:refnum<visa-resource-name>, error out=w697:errorcluster)  [unwired: 1 out]
              }
              frame #3 {
                n327 = Wait (ms)(milliseconds to wait=u32 50) -> ()  [unwired: 1 out]
              }
            }
            n328 = VISA Clear(VISA resource name=w680, error in (no error)=w682) -> (VISA resource name out=w678:refnum<visa-resource-name>, error out=w679:errorcluster)
          }
        }
        n329 = local write "VISA resource name out"(w644) -> ()
      }
      event "F-R VISAR1": Value Change {
        w719 = u16 0 items=["T0"=0, "A"=2, "B"=3, "C"=4, "D"=5, "E"=6, "F"=7, "G"=8, "H"=9] ("Reference Channel (0:T0)")
        w723 = u16 2 items=["A"=2, "B"=3, "C"=4, "D"=5, "E"=6, "F"=7, "G"=8, "H"=9] ("Channel to Modify (2:A)")
        n330 = event-data() -> ()  [unwired: 1 in, 6 out]
        n331 = Subtract(x="Delay A (0 s)", y=ext 100.0) -> (x-y=w706:ext)
        n332 = Divide(x=w706, y=ext 1000000000.0) -> (x/y=w709:ext)
        n333 = Format Into String(format string="%.;DLAY%d,%d,%.12g" ("Set Delay Command"), w723, w719, w709) -> (resulting string=w722:string)  [unwired: 2 in, 1 out]
        n334 = Concatenate Strings(w722, "\r\n") -> (w721:string)
        n335 = flat-sequence {
          tunnel: w721 -> [w729]
          tunnel: w718 -> [w728]
          tunnel: refnum<visa-resource-name> "DG645" ("VISA resource name") -> [w727]
          tunnel: [w726] -> w713
          tunnel: [w725] -> w712
          tunnel: [w731] -> w714
          tunnel: [w732] -> w716
          tunnel: w713 -> [w732]
          tunnel: w712 -> [w731]
          frame #0 {
            n336 = VISA Write(VISA resource name=w727, write buffer=w729, error in (no error)=w728) -> (VISA resource name out=w725:refnum<visa-resource-name>, error out=w726:errorcluster)  [unwired: 1 out]
          }
          frame #1 {
            n337 = Wait (ms)(milliseconds to wait=u32 50) -> ()  [unwired: 1 out]
          }
        }
        n338 = VISA Clear(VISA resource name=w714, error in (no error)=w716) -> (VISA resource name out=w711:refnum<visa-resource-name>, error out=w715:errorcluster)
        n339 = local write "VISA resource name out"(w711) -> ()
      }
      event "F-R VISAR2": Value Change {
        w746 = u16 0 items=["T0"=0, "A"=2, "B"=3, "C"=4, "D"=5, "E"=6, "F"=7, "G"=8, "H"=9] ("Reference Channel (0:T0)")
        w750 = u16 3 items=["A"=2, "B"=3, "C"=4, "D"=5, "E"=6, "F"=7, "G"=8, "H"=9] ("Channel to Modify (2:A)")
        n340 = event-data() -> ()  [unwired: 1 in, 6 out]
        n341 = Subtract(x="Delay B (0 s)", y=ext 100.0) -> (x-y=w733:ext)
        n342 = Divide(x=w733, y=ext 1000000000.0) -> (x/y=w736:ext)
        n343 = Format Into String(format string="%.;DLAY%d,%d,%.12g" ("Set Delay Command"), w750, w746, w736) -> (resulting string=w749:string)  [unwired: 2 in, 1 out]
        n344 = Concatenate Strings(w749, "\r\n") -> (w748:string)
        n345 = flat-sequence {
          tunnel: w748 -> [w756]
          tunnel: w745 -> [w755]
          tunnel: refnum<visa-resource-name> "DG645" ("VISA resource name") -> [w754]
          tunnel: [w753] -> w740
          tunnel: [w752] -> w739
          tunnel: [w758] -> w741
          tunnel: [w759] -> w743
          tunnel: w740 -> [w759]
          tunnel: w739 -> [w758]
          frame #0 {
            n346 = VISA Write(VISA resource name=w754, write buffer=w756, error in (no error)=w755) -> (VISA resource name out=w752:refnum<visa-resource-name>, error out=w753:errorcluster)  [unwired: 1 out]
          }
          frame #1 {
            n347 = Wait (ms)(milliseconds to wait=u32 50) -> ()  [unwired: 1 out]
          }
        }
        n348 = VISA Clear(VISA resource name=w741, error in (no error)=w743) -> (VISA resource name out=w738:refnum<visa-resource-name>, error out=w742:errorcluster)
        n349 = local write "VISA resource name out"(w738) -> ()
      }
      event "FI": Value Change {
        w773 = u16 0 items=["T0"=0, "A"=2, "B"=3, "C"=4, "D"=5, "E"=6, "F"=7, "G"=8, "H"=9] ("Reference Channel (0:T0)")
        w777 = u16 4 items=["A"=2, "B"=3, "C"=4, "D"=5, "E"=6, "F"=7, "G"=8, "H"=9] ("Channel to Modify (2:A)")
        n350 = event-data() -> ()  [unwired: 1 in, 6 out]
        n351 = Subtract(x="Delay C (0 s)", y=ext 100.0) -> (x-y=w761:ext)
        n352 = Divide(x=w761, y=ext 1000000000.0) -> (x/y=w762:ext)
        n353 = Format Into String(format string="%.;DLAY%d,%d,%.12g" ("Set Delay Command"), w777, w773, w762) -> (resulting string=w776:string)  [unwired: 2 in, 1 out]
        n354 = Concatenate Strings(w776, "\r\n") -> (w775:string)
        n355 = flat-sequence {
          tunnel: w775 -> [w783]
          tunnel: w772 -> [w782]
          tunnel: refnum<visa-resource-name> "DG645" ("VISA resource name") -> [w781]
          tunnel: [w780] -> w767
          tunnel: [w779] -> w766
          tunnel: [w785] -> w768
          tunnel: [w786] -> w769
          tunnel: w767 -> [w786]
          tunnel: w766 -> [w785]
          frame #0 {
            n356 = VISA Write(VISA resource name=w781, write buffer=w783, error in (no error)=w782) -> (VISA resource name out=w779:refnum<visa-resource-name>, error out=w780:errorcluster)  [unwired: 1 out]
          }
          frame #1 {
            n357 = Wait (ms)(milliseconds to wait=u32 50) -> ()  [unwired: 1 out]
          }
        }
        n358 = VISA Clear(VISA resource name=w768, error in (no error)=w769) -> (VISA resource name out=w765:refnum<visa-resource-name>, error out=w770:errorcluster)
        n359 = local write "VISA resource name out"(w765) -> ()
      }
      event "GF": Value Change {
        w800 = u16 0 items=["T0"=0, "A"=2, "B"=3, "C"=4, "D"=5, "E"=6, "F"=7, "G"=8, "H"=9] ("Reference Channel (0:T0)")
        w804 = u16 5 items=["A"=2, "B"=3, "C"=4, "D"=5, "E"=6, "F"=7, "G"=8, "H"=9] ("Channel to Modify (2:A)")
        n360 = event-data() -> ()  [unwired: 1 in, 6 out]
        n361 = Subtract(x="Delay D (0 s)", y=ext 100.0) -> (x-y=w789:ext)
        n362 = Divide(x=w789, y=ext 1000000000.0) -> (x/y=w787:ext)
        n363 = Format Into String(format string="%.;DLAY%d,%d,%.12g" ("Set Delay Command"), w804, w800, w787) -> (resulting string=w803:string)  [unwired: 2 in, 1 out]
        n364 = Concatenate Strings(w803, "\r\n") -> (w802:string)
        n365 = flat-sequence {
          tunnel: w802 -> [w810]
          tunnel: w799 -> [w809]
          tunnel: refnum<visa-resource-name> "DG645" ("VISA resource name") -> [w808]
          tunnel: [w807] -> w794
          tunnel: [w806] -> w793
          tunnel: [w812] -> w795
          tunnel: [w813] -> w797
          tunnel: w794 -> [w813]
          tunnel: w793 -> [w812]
          frame #0 {
            n366 = VISA Write(VISA resource name=w808, write buffer=w810, error in (no error)=w809) -> (VISA resource name out=w806:refnum<visa-resource-name>, error out=w807:errorcluster)  [unwired: 1 out]
          }
          frame #1 {
            n367 = Wait (ms)(milliseconds to wait=u32 50) -> ()  [unwired: 1 out]
          }
        }
        n368 = VISA Clear(VISA resource name=w795, error in (no error)=w797) -> (VISA resource name out=w792:refnum<visa-resource-name>, error out=w796:errorcluster)
        n369 = local write "VISA resource name out"(w792) -> ()
      }
      event "Kamera Y": Value Change {
        w827 = u16 0 items=["T0"=0, "A"=2, "B"=3, "C"=4, "D"=5, "E"=6, "F"=7, "G"=8, "H"=9] ("Reference Channel (0:T0)")
        w831 = u16 6 items=["A"=2, "B"=3, "C"=4, "D"=5, "E"=6, "F"=7, "G"=8, "H"=9] ("Channel to Modify (2:A)")
        n370 = event-data() -> ()  [unwired: 1 in, 6 out]
        n371 = Subtract(x="Delay E (0 s)", y=ext 100.0) -> (x-y=w815:ext)
        n372 = Divide(x=w815, y=ext 1000000000.0) -> (x/y=w814:ext)
        n373 = Format Into String(format string="%.;DLAY%d,%d,%.12g" ("Set Delay Command"), w831, w827, w814) -> (resulting string=w830:string)  [unwired: 2 in, 1 out]
        n374 = Concatenate Strings(w830, "\r\n") -> (w829:string)
        n375 = flat-sequence {
          tunnel: w829 -> [w837]
          tunnel: w826 -> [w836]
          tunnel: refnum<visa-resource-name> "DG645" ("VISA resource name") -> [w835]
          tunnel: [w834] -> w821
          tunnel: [w833] -> w820
          tunnel: [w839] -> w822
          tunnel: [w840] -> w824
          tunnel: w821 -> [w840]
          tunnel: w820 -> [w839]
          frame #0 {
            n376 = VISA Write(VISA resource name=w835, write buffer=w837, error in (no error)=w836) -> (VISA resource name out=w833:refnum<visa-resource-name>, error out=w834:errorcluster)  [unwired: 1 out]
          }
          frame #1 {
            n377 = Wait (ms)(milliseconds to wait=u32 50) -> ()  [unwired: 1 out]
          }
        }
        n378 = VISA Clear(VISA resource name=w822, error in (no error)=w824) -> (VISA resource name out=w819:refnum<visa-resource-name>, error out=w823:errorcluster)
        n379 = local write "VISA resource name out"(w819) -> ()
      }
      event "BK1": Value Change {
        w854 = u16 0 items=["T0"=0, "A"=2, "B"=3, "C"=4, "D"=5, "E"=6, "F"=7, "G"=8, "H"=9] ("Reference Channel (0:T0)")
        w858 = u16 7 items=["A"=2, "B"=3, "C"=4, "D"=5, "E"=6, "F"=7, "G"=8, "H"=9] ("Channel to Modify (2:A)")
        n380 = event-data() -> ()  [unwired: 1 in, 6 out]
        n381 = Subtract(x="Delay F (0 s)", y=ext 100.0) -> (x-y=w842:ext)
        n382 = Divide(x=w842, y=ext 1000000000.0) -> (x/y=w841:ext)
        n383 = Format Into String(format string="%.;DLAY%d,%d,%.12g" ("Set Delay Command"), w858, w854, w841) -> (resulting string=w857:string)  [unwired: 2 in, 1 out]
        n384 = Concatenate Strings(w857, "\r\n") -> (w856:string)
        n385 = flat-sequence {
          tunnel: w856 -> [w864]
          tunnel: w853 -> [w863]
          tunnel: refnum<visa-resource-name> "DG645" ("VISA resource name") -> [w862]
          tunnel: [w861] -> w848
          tunnel: [w860] -> w847
          tunnel: [w866] -> w850
          tunnel: [w867] -> w851
          tunnel: w848 -> [w867]
          tunnel: w847 -> [w866]
          frame #0 {
            n386 = VISA Write(VISA resource name=w862, write buffer=w864, error in (no error)=w863) -> (VISA resource name out=w860:refnum<visa-resource-name>, error out=w861:errorcluster)  [unwired: 1 out]
          }
          frame #1 {
            n387 = Wait (ms)(milliseconds to wait=u32 50) -> ()  [unwired: 1 out]
          }
        }
        n388 = VISA Clear(VISA resource name=w850, error in (no error)=w851) -> (VISA resource name out=w846:refnum<visa-resource-name>, error out=w849:errorcluster)
        n389 = local write "VISA resource name out"(w846) -> ()
      }
      event "BK2": Value Change {
        w881 = u16 0 items=["T0"=0, "A"=2, "B"=3, "C"=4, "D"=5, "E"=6, "F"=7, "G"=8, "H"=9] ("Reference Channel (0:T0)")
        w885 = u16 8 items=["A"=2, "B"=3, "C"=4, "D"=5, "E"=6, "F"=7, "G"=8, "H"=9] ("Channel to Modify (2:A)")
        n390 = event-data() -> ()  [unwired: 1 in, 6 out]
        n391 = Subtract(x="Delay G (0 s)", y=ext 100.0) -> (x-y=w869:ext)
        n392 = Divide(x=w869, y=ext 1000000000.0) -> (x/y=w868:ext)
        n393 = Format Into String(format string="%.;DLAY%d,%d,%.12g" ("Set Delay Command"), w885, w881, w868) -> (resulting string=w884:string)  [unwired: 2 in, 1 out]
        n394 = Concatenate Strings(w884, "\r\n") -> (w883:string)
        n395 = flat-sequence {
          tunnel: w883 -> [w891]
          tunnel: w880 -> [w890]
          tunnel: refnum<visa-resource-name> "DG645" ("VISA resource name") -> [w889]
          tunnel: [w888] -> w875
          tunnel: [w887] -> w874
          tunnel: [w893] -> w876
          tunnel: [w894] -> w878
          tunnel: w875 -> [w894]
          tunnel: w874 -> [w893]
          frame #0 {
            n396 = VISA Write(VISA resource name=w889, write buffer=w891, error in (no error)=w890) -> (VISA resource name out=w887:refnum<visa-resource-name>, error out=w888:errorcluster)  [unwired: 1 out]
          }
          frame #1 {
            n397 = Wait (ms)(milliseconds to wait=u32 50) -> ()  [unwired: 1 out]
          }
        }
        n398 = VISA Clear(VISA resource name=w876, error in (no error)=w878) -> (VISA resource name out=w873:refnum<visa-resource-name>, error out=w877:errorcluster)
        n399 = local write "VISA resource name out"(w873) -> ()
      }
      event "BK3": Value Change {
        w908 = u16 0 items=["T0"=0, "A"=2, "B"=3, "C"=4, "D"=5, "E"=6, "F"=7, "G"=8, "H"=9] ("Reference Channel (0:T0)")
        w912 = u16 9 items=["A"=2, "B"=3, "C"=4, "D"=5, "E"=6, "F"=7, "G"=8, "H"=9] ("Channel to Modify (2:A)")
        n400 = event-data() -> ()  [unwired: 1 in, 6 out]
        n401 = Subtract(x="Delay H (0 s)", y=ext 100.0) -> (x-y=w896:ext)
        n402 = Divide(x=w896, y=ext 1000000000.0) -> (x/y=w895:ext)
        n403 = Format Into String(format string="%.;DLAY%d,%d,%.12g" ("Set Delay Command"), w912, w908, w895) -> (resulting string=w911:string)  [unwired: 2 in, 1 out]
        n404 = Concatenate Strings(w911, "\r\n") -> (w910:string)
        n405 = flat-sequence {
          tunnel: w910 -> [w918]
          tunnel: w907 -> [w917]
          tunnel: refnum<visa-resource-name> "DG645" ("VISA resource name") -> [w916]
          tunnel: [w915] -> w902
          tunnel: [w914] -> w901
          tunnel: [w920] -> w903
          tunnel: [w921] -> w905
          tunnel: w902 -> [w921]
          tunnel: w901 -> [w920]
          frame #0 {
            n406 = VISA Write(VISA resource name=w916, write buffer=w918, error in (no error)=w917) -> (VISA resource name out=w914:refnum<visa-resource-name>, error out=w915:errorcluster)  [unwired: 1 out]
          }
          frame #1 {
            n407 = Wait (ms)(milliseconds to wait=u32 50) -> ()  [unwired: 1 out]
          }
        }
        n408 = VISA Clear(VISA resource name=w903, error in (no error)=w905) -> (VISA resource name out=w900:refnum<visa-resource-name>, error out=w904:errorcluster)
        n409 = local write "VISA resource name out"(w900) -> ()
      }
      event "BZ2K1W": Value Change {
        n410 = event-data() -> ("NewVal"=w930:bool)  [unwired: 1 in]
        n411 = flat-sequence {
          tunnel: w930 -> [w935]
          tunnel: w929 -> [w934]
          tunnel: refnum<visa-resource-name> "Adam" ("VISA resource name") -> [w933]
          tunnel: [w932] -> w924
          tunnel: [w931] -> w923
          tunnel: [w951] -> w926
          tunnel: [w952] -> w927
          tunnel: w924 -> [w952]
          tunnel: w923 -> [w951]
          frame #0 {
            n412 = case shown="True" w935 {
              tunnel: [w939 w946] -> w931
              tunnel: [w938 w945] -> w932
              tunnel: w934 -> [w937 w944]
              tunnel: w933 -> [w936 w943]
              frame False {
                n413 = Concatenate Strings("#041000" ("string"), "\r\n") -> (w942:string)
                n414 = VISA Write(VISA resource name=w936, write buffer=w942, error in (no error)=w937) -> (VISA resource name out=w939:refnum<visa-resource-name>, error out=w938:errorcluster)  [unwired: 1 out]
              }
              frame True {
                n415 = Concatenate Strings("#041001" ("string"), "\r\n") -> (w949:string)
                n416 = VISA Write(VISA resource name=w943, write buffer=w949, error in (no error)=w944) -> (VISA resource name out=w946:refnum<visa-resource-name>, error out=w945:errorcluster)  [unwired: 1 out]
              }
            }
          }
          frame #1 {
            n417 = Wait (ms)(milliseconds to wait=u32 50) -> ()  [unwired: 1 out]
          }
        }
        n418 = VISA Clear(VISA resource name=w926, error in (no error)=w927) -> (VISA resource name out=w922:refnum<visa-resource-name>, error out=w925:errorcluster)
        n419 = local write "VISA resource name out"(w922) -> ()
      }
      event "DZ1K2W": Value Change {
        n420 = event-data() -> ("NewVal"=w959:bool)  [unwired: 1 in]
        n421 = flat-sequence {
          tunnel: w959 -> [w964]
          tunnel: refnum<visa-resource-name> "Adam" ("VISA resource name") -> [w963]
          tunnel: w957 -> [w962]
          tunnel: [w966] -> w955
          tunnel: [w965] -> w954
          tunnel: [w982] -> w960
          tunnel: [w983] -> w961
          tunnel: w955 -> [w983]
          tunnel: w954 -> [w982]
          frame #0 {
            n422 = case shown="True" w964 {
              tunnel: [w970 w977] -> w966
              tunnel: [w969 w976] -> w965
              tunnel: w962 -> [w968 w975]
              tunnel: w963 -> [w967 w974]
              frame False {
                n423 = Concatenate Strings("#041100" ("string"), "\r\n") -> (w973:string)
                n424 = VISA Write(VISA resource name=w967, write buffer=w973, error in (no error)=w968) -> (VISA resource name out=w969:refnum<visa-resource-name>, error out=w970:errorcluster)  [unwired: 1 out]
              }
              frame True {
                n425 = Concatenate Strings("#041101" ("string"), "\r\n") -> (w980:string)
                n426 = VISA Write(VISA resource name=w974, write buffer=w980, error in (no error)=w975) -> (VISA resource name out=w976:refnum<visa-resource-name>, error out=w977:errorcluster)  [unwired: 1 out]
              }
            }
          }
          frame #1 {
            n427 = Wait (ms)(milliseconds to wait=u32 50) -> ()  [unwired: 1 out]
          }
        }
        n428 = VISA Clear(VISA resource name=w960, error in (no error)=w961) -> (VISA resource name out=w953:refnum<visa-resource-name>, error out=w956:errorcluster)
        n429 = local write "VISA resource name out"(w953) -> ()
      }
      event "DZ2K2W": Value Change {
        n430 = event-data() -> ("NewVal"=w992:bool)  [unwired: 1 in]
        n431 = flat-sequence {
          tunnel: w992 -> [w997]
          tunnel: refnum<visa-resource-name> "Adam" ("VISA resource name") -> [w996]
          tunnel: w990 -> [w995]
          tunnel: [w994] -> w986
          tunnel: [w993] -> w985
          tunnel: [w1013] -> w988
          tunnel: [w1014] -> w989
          tunnel: w986 -> [w1014]
          tunnel: w985 -> [w1013]
          frame #0 {
            n432 = case shown="True" w997 {
              tunnel: [w999 w1008] -> w994
              tunnel: [w998 w1007] -> w993
              tunnel: w996 -> [w1001 w1006]
              tunnel: w995 -> [w1000 w1005]
              frame False {
                n433 = Concatenate Strings("#041200" ("string"), "\r\n") -> (w1004:string)
                n434 = VISA Write(VISA resource name=w1001, write buffer=w1004, error in (no error)=w1000) -> (VISA resource name out=w998:refnum<visa-resource-name>, error out=w999:errorcluster)  [unwired: 1 out]
              }
              frame True {
                n435 = Concatenate Strings("#041201" ("string"), "\r\n") -> (w1011:string)
                n436 = VISA Write(VISA resource name=w1006, write buffer=w1011, error in (no error)=w1005) -> (VISA resource name out=w1007:refnum<visa-resource-name>, error out=w1008:errorcluster)  [unwired: 1 out]
              }
            }
          }
          frame #1 {
            n437 = Wait (ms)(milliseconds to wait=u32 50) -> ()  [unwired: 1 out]
          }
        }
        n438 = VISA Clear(VISA resource name=w988, error in (no error)=w989) -> (VISA resource name out=w984:refnum<visa-resource-name>, error out=w987:errorcluster)
        n439 = local write "VISA resource name out"(w984) -> ()
      }
      event "BZ1K2W": Value Change {
        n440 = event-data() -> ("NewVal"=w1023:bool)  [unwired: 1 in]
        n441 = flat-sequence {
          tunnel: w1023 -> [w1028]
          tunnel: refnum<visa-resource-name> "Adam" ("VISA resource name") -> [w1027]
          tunnel: w1021 -> [w1026]
          tunnel: [w1025] -> w1017
          tunnel: [w1024] -> w1016
          tunnel: [w1044] -> w1019
          tunnel: [w1045] -> w1020
          tunnel: w1017 -> [w1045]
          tunnel: w1016 -> [w1044]
          frame #0 {
            n442 = case shown="True" w1028 {
              tunnel: w1027 -> [w1032 w1039]
              tunnel: w1026 -> [w1031 w1038]
              tunnel: [w1030 w1036] -> w1025
              tunnel: [w1029 w1037] -> w1024
              frame False {
                n443 = Concatenate Strings("#041300" ("string"), "\r\n") -> (w1035:string)
                n444 = VISA Write(VISA resource name=w1032, write buffer=w1035, error in (no error)=w1031) -> (VISA resource name out=w1029:refnum<visa-resource-name>, error out=w1030:errorcluster)  [unwired: 1 out]
              }
              frame True {
                n445 = Concatenate Strings("#041301" ("string"), "\r\n") -> (w1042:string)
                n446 = VISA Write(VISA resource name=w1039, write buffer=w1042, error in (no error)=w1038) -> (VISA resource name out=w1037:refnum<visa-resource-name>, error out=w1036:errorcluster)  [unwired: 1 out]
              }
            }
          }
          frame #1 {
            n447 = Wait (ms)(milliseconds to wait=u32 50) -> ()  [unwired: 1 out]
          }
        }
        n448 = VISA Clear(VISA resource name=w1019, error in (no error)=w1020) -> (VISA resource name out=w1015:refnum<visa-resource-name>, error out=w1018:errorcluster)
        n449 = local write "VISA resource name out"(w1015) -> ()
      }
      event "BZ2K2W": Value Change {
        n450 = event-data() -> ("NewVal"=w1054:bool)  [unwired: 1 in]
        n451 = flat-sequence {
          tunnel: w1054 -> [w1059]
          tunnel: refnum<visa-resource-name> "Adam" ("VISA resource name") -> [w1058]
          tunnel: w1052 -> [w1057]
          tunnel: [w1056] -> w1048
          tunnel: [w1055] -> w1047
          tunnel: [w1075] -> w1049
          tunnel: [w1076] -> w1051
          tunnel: w1048 -> [w1076]
          tunnel: w1047 -> [w1075]
          frame #0 {
            n452 = case shown="True" w1059 {
              tunnel: [w1061 w1070] -> w1056
              tunnel: [w1060 w1069] -> w1055
              tunnel: w1057 -> [w1063 w1068]
              tunnel: w1058 -> [w1062 w1067]
              frame False {
                n453 = Concatenate Strings("#041400" ("string"), "\r\n") -> (w1066:string)
                n454 = VISA Write(VISA resource name=w1062, write buffer=w1066, error in (no error)=w1063) -> (VISA resource name out=w1060:refnum<visa-resource-name>, error out=w1061:errorcluster)  [unwired: 1 out]
              }
              frame True {
                n455 = Concatenate Strings("#041401" ("string"), "\r\n") -> (w1073:string)
                n456 = VISA Write(VISA resource name=w1067, write buffer=w1073, error in (no error)=w1068) -> (VISA resource name out=w1069:refnum<visa-resource-name>, error out=w1070:errorcluster)  [unwired: 1 out]
              }
            }
          }
          frame #1 {
            n457 = Wait (ms)(milliseconds to wait=u32 50) -> ()  [unwired: 1 out]
          }
        }
        n458 = VISA Clear(VISA resource name=w1049, error in (no error)=w1051) -> (VISA resource name out=w1046:refnum<visa-resource-name>, error out=w1050:errorcluster)
        n459 = local write "VISA resource name out"(w1046) -> ()
      }
      event "DZ1K1W": Value Change {
        n460 = event-data() -> ("NewVal"=w1085:bool)  [unwired: 1 in]
        n461 = flat-sequence {
          tunnel: w1085 -> [w1090]
          tunnel: refnum<visa-resource-name> "Adam" ("VISA resource name") -> [w1089]
          tunnel: w1083 -> [w1088]
          tunnel: [w1087] -> w1079
          tunnel: [w1086] -> w1078
          tunnel: [w1106] -> w1081
          tunnel: [w1107] -> w1082
          tunnel: w1079 -> [w1107]
          tunnel: w1078 -> [w1106]
          frame #0 {
            n462 = case shown="True" w1090 {
              tunnel: [w1094 w1101] -> w1087
              tunnel: [w1093 w1100] -> w1086
              tunnel: w1089 -> [w1092 w1098]
              tunnel: w1088 -> [w1091 w1099]
              frame False {
                n463 = Concatenate Strings("#041500" ("string"), "\r\n") -> (w1097:string)
                n464 = VISA Write(VISA resource name=w1092, write buffer=w1097, error in (no error)=w1091) -> (VISA resource name out=w1093:refnum<visa-resource-name>, error out=w1094:errorcluster)  [unwired: 1 out]
              }
              frame True {
                n465 = Concatenate Strings("#041501" ("string"), "\r\n") -> (w1104:string)
                n466 = VISA Write(VISA resource name=w1098, write buffer=w1104, error in (no error)=w1099) -> (VISA resource name out=w1100:refnum<visa-resource-name>, error out=w1101:errorcluster)  [unwired: 1 out]
              }
            }
          }
          frame #1 {
            n467 = Wait (ms)(milliseconds to wait=u32 50) -> ()  [unwired: 1 out]
          }
        }
        n468 = VISA Clear(VISA resource name=w1081, error in (no error)=w1082) -> (VISA resource name out=w1077:refnum<visa-resource-name>, error out=w1080:errorcluster)
        n469 = local write "VISA resource name out"(w1077) -> ()
      }
      event "DZ2K1W": Value Change {
        n470 = event-data() -> ("NewVal"=w1116:bool)  [unwired: 1 in]
        n471 = flat-sequence {
          tunnel: w1116 -> [w1121]
          tunnel: refnum<visa-resource-name> "Adam" ("VISA resource name") -> [w1120]
          tunnel: w1114 -> [w1119]
          tunnel: [w1118] -> w1110
          tunnel: [w1117] -> w1109
          tunnel: [w1137] -> w1111
          tunnel: [w1138] -> w1113
          tunnel: w1110 -> [w1138]
          tunnel: w1109 -> [w1137]
          frame #0 {
            n472 = case shown="True" w1121 {
              tunnel: [w1125 w1131] -> w1118
              tunnel: [w1124 w1132] -> w1117
              tunnel: w1119 -> [w1123 w1130]
              tunnel: w1120 -> [w1122 w1129]
              frame False {
                n473 = Concatenate Strings("#041600" ("string"), "\r\n") -> (w1128:string)
                n474 = VISA Write(VISA resource name=w1122, write buffer=w1128, error in (no error)=w1123) -> (VISA resource name out=w1124:refnum<visa-resource-name>, error out=w1125:errorcluster)  [unwired: 1 out]
              }
              frame True {
                n475 = Concatenate Strings("#041601" ("string"), "\r\n") -> (w1135:string)
                n476 = VISA Write(VISA resource name=w1129, write buffer=w1135, error in (no error)=w1130) -> (VISA resource name out=w1132:refnum<visa-resource-name>, error out=w1131:errorcluster)  [unwired: 1 out]
              }
            }
          }
          frame #1 {
            n477 = Wait (ms)(milliseconds to wait=u32 50) -> ()  [unwired: 1 out]
          }
        }
        n478 = VISA Clear(VISA resource name=w1111, error in (no error)=w1113) -> (VISA resource name out=w1108:refnum<visa-resource-name>, error out=w1112:errorcluster)
        n479 = local write "VISA resource name out"(w1108) -> ()
      }
      event "BZ1K1W": Value Change {
        n480 = event-data() -> ("NewVal"=w1147:bool)  [unwired: 1 in]
        n481 = flat-sequence {
          tunnel: w1147 -> [w1152]
          tunnel: refnum<visa-resource-name> "Adam" ("VISA resource name") -> [w1151]
          tunnel: w1145 -> [w1150]
          tunnel: [w1149] -> w1141
          tunnel: [w1148] -> w1140
          tunnel: [w1168] -> w1143
          tunnel: [w1169] -> w1144
          tunnel: w1141 -> [w1169]
          tunnel: w1140 -> [w1168]
          frame #0 {
            n482 = case shown="True" w1152 {
              tunnel: w1150 -> [w1156 w1160]
              tunnel: w1151 -> [w1155 w1161]
              tunnel: [w1154 w1163] -> w1149
              tunnel: [w1153 w1162] -> w1148
              frame False {
                n483 = Concatenate Strings("#041700" ("string"), "\r\n") -> (w1159:string)
                n484 = VISA Write(VISA resource name=w1155, write buffer=w1159, error in (no error)=w1156) -> (VISA resource name out=w1153:refnum<visa-resource-name>, error out=w1154:errorcluster)  [unwired: 1 out]
              }
              frame True {
                n485 = Concatenate Strings("#041701" ("string"), "\r\n") -> (w1166:string)
                n486 = VISA Write(VISA resource name=w1161, write buffer=w1166, error in (no error)=w1160) -> (VISA resource name out=w1162:refnum<visa-resource-name>, error out=w1163:errorcluster)  [unwired: 1 out]
              }
            }
          }
          frame #1 {
            n487 = Wait (ms)(milliseconds to wait=u32 50) -> ()  [unwired: 1 out]
          }
        }
        n488 = VISA Clear(VISA resource name=w1143, error in (no error)=w1144) -> (VISA resource name out=w1139:refnum<visa-resource-name>, error out=w1142:errorcluster)
        n489 = local write "VISA resource name out"(w1139) -> ()
      }
      event "GF": Value Change {
        n490 = event-data() -> ("NewVal"=w1178:bool)  [unwired: 1 in]
        n491 = flat-sequence {
          tunnel: w1178 -> [w1183]
          tunnel: refnum<visa-resource-name> "Adam" ("VISA resource name") -> [w1182]
          tunnel: w1176 -> [w1181]
          tunnel: [w1180] -> w1172
          tunnel: [w1179] -> w1171
          tunnel: [w1199] -> w1174
          tunnel: [w1200] -> w1175
          tunnel: w1172 -> [w1200]
          tunnel: w1171 -> [w1199]
          frame #0 {
            n492 = case shown="True" w1183 {
              tunnel: [w1187 w1194] -> w1179
              tunnel: [w1186 w1193] -> w1180
              tunnel: w1181 -> [w1185 w1192]
              tunnel: w1182 -> [w1184 w1191]
              frame False {
                n493 = Concatenate Strings("#051000" ("string"), "\r\n") -> (w1190:string)
                n494 = VISA Write(VISA resource name=w1184, write buffer=w1190, error in (no error)=w1185) -> (VISA resource name out=w1187:refnum<visa-resource-name>, error out=w1186:errorcluster)  [unwired: 1 out]
              }
              frame True {
                n495 = Concatenate Strings("#051001" ("string"), "\r\n") -> (w1197:string)
                n496 = VISA Write(VISA resource name=w1191, write buffer=w1197, error in (no error)=w1192) -> (VISA resource name out=w1194:refnum<visa-resource-name>, error out=w1193:errorcluster)  [unwired: 1 out]
              }
            }
          }
          frame #1 {
            n497 = Wait (ms)(milliseconds to wait=u32 50) -> ()  [unwired: 1 out]
          }
        }
        n498 = VISA Clear(VISA resource name=w1174, error in (no error)=w1175) -> (VISA resource name out=w1170:refnum<visa-resource-name>, error out=w1173:errorcluster)
        n499 = local write "VISA resource name out"(w1170) -> ()
      }
      event "Kamera Y": Value Change {
        n500 = event-data() -> ("NewVal"=w1209:bool)  [unwired: 1 in]
        n501 = flat-sequence {
          tunnel: w1209 -> [w1214]
          tunnel: w1208 -> [w1213]
          tunnel: refnum<visa-resource-name> "Adam" ("VISA resource name") -> [w1212]
          tunnel: [w1211] -> w1203
          tunnel: [w1210] -> w1202
          tunnel: [w1230] -> w1205
          tunnel: [w1231] -> w1206
          tunnel: w1203 -> [w1231]
          tunnel: w1202 -> [w1230]
          frame #0 {
            n502 = case shown="True" w1214 {
              tunnel: [w1218 w1225] -> w1211
              tunnel: [w1217 w1224] -> w1210
              tunnel: w1213 -> [w1216 w1223]
              tunnel: w1212 -> [w1215 w1222]
              frame False {
                n503 = Concatenate Strings("#051100" ("string"), "\r\n") -> (w1221:string)
                n504 = VISA Write(VISA resource name=w1215, write buffer=w1221, error in (no error)=w1216) -> (VISA resource name out=w1217:refnum<visa-resource-name>, error out=w1218:errorcluster)  [unwired: 1 out]
              }
              frame True {
                n505 = Concatenate Strings("#051101" ("string"), "\r\n") -> (w1228:string)
                n506 = VISA Write(VISA resource name=w1222, write buffer=w1228, error in (no error)=w1223) -> (VISA resource name out=w1224:refnum<visa-resource-name>, error out=w1225:errorcluster)  [unwired: 1 out]
              }
            }
          }
          frame #1 {
            n507 = Wait (ms)(milliseconds to wait=u32 50) -> ()  [unwired: 1 out]
          }
        }
        n508 = VISA Clear(VISA resource name=w1205, error in (no error)=w1206) -> (VISA resource name out=w1201:refnum<visa-resource-name>, error out=w1204:errorcluster)
        n509 = local write "VISA resource name out"(w1201) -> ()
      }
      event "BK1": Value Change {
        n510 = event-data() -> ("NewVal"=w1240:bool)  [unwired: 1 in]
        n511 = flat-sequence {
          tunnel: w1240 -> [w1245]
          tunnel: refnum<visa-resource-name> "Adam" ("VISA resource name") -> [w1244]
          tunnel: w1238 -> [w1243]
          tunnel: [w1242] -> w1234
          tunnel: [w1241] -> w1233
          tunnel: [w1261] -> w1236
          tunnel: [w1262] -> w1237
          tunnel: w1234 -> [w1262]
          tunnel: w1233 -> [w1261]
          frame #0 {
            n512 = case shown="True" w1245 {
              tunnel: [w1247 w1256] -> w1242
              tunnel: [w1246 w1255] -> w1241
              tunnel: w1244 -> [w1249 w1254]
              tunnel: w1243 -> [w1248 w1253]
              frame False {
                n513 = Concatenate Strings("#051200" ("string"), "\r\n") -> (w1252:string)
                n514 = VISA Write(VISA resource name=w1249, write buffer=w1252, error in (no error)=w1248) -> (VISA resource name out=w1246:refnum<visa-resource-name>, error out=w1247:errorcluster)  [unwired: 1 out]
              }
              frame True {
                n515 = Concatenate Strings("#051201" ("string"), "\r\n") -> (w1259:string)
                n516 = VISA Write(VISA resource name=w1254, write buffer=w1259, error in (no error)=w1253) -> (VISA resource name out=w1255:refnum<visa-resource-name>, error out=w1256:errorcluster)  [unwired: 1 out]
              }
            }
          }
          frame #1 {
            n517 = Wait (ms)(milliseconds to wait=u32 50) -> ()  [unwired: 1 out]
          }
        }
        n518 = VISA Clear(VISA resource name=w1236, error in (no error)=w1237) -> (VISA resource name out=w1232:refnum<visa-resource-name>, error out=w1235:errorcluster)
        n519 = local write "VISA resource name out"(w1232) -> ()
      }
      event "BK 2": Value Change {
        n520 = event-data() -> ("NewVal"=w1271:bool)  [unwired: 1 in]
        n521 = flat-sequence {
          tunnel: w1271 -> [w1276]
          tunnel: refnum<visa-resource-name> "Adam" ("VISA resource name") -> [w1275]
          tunnel: w1269 -> [w1274]
          tunnel: [w1273] -> w1265
          tunnel: [w1272] -> w1264
          tunnel: [w1292] -> w1267
          tunnel: [w1293] -> w1268
          tunnel: w1265 -> [w1293]
          tunnel: w1264 -> [w1292]
          frame #0 {
            n522 = case shown="True" w1276 {
              tunnel: w1275 -> [w1280 w1287]
              tunnel: w1274 -> [w1279 w1286]
              tunnel: [w1278 w1284] -> w1273
              tunnel: [w1277 w1285] -> w1272
              frame False {
                n523 = Concatenate Strings("#051300" ("string"), "\r\n") -> (w1283:string)
                n524 = VISA Write(VISA resource name=w1280, write buffer=w1283, error in (no error)=w1279) -> (VISA resource name out=w1277:refnum<visa-resource-name>, error out=w1278:errorcluster)  [unwired: 1 out]
              }
              frame True {
                n525 = Concatenate Strings("#051301" ("string"), "\r\n") -> (w1290:string)
                n526 = VISA Write(VISA resource name=w1287, write buffer=w1290, error in (no error)=w1286) -> (VISA resource name out=w1285:refnum<visa-resource-name>, error out=w1284:errorcluster)  [unwired: 1 out]
              }
            }
          }
          frame #1 {
            n527 = Wait (ms)(milliseconds to wait=u32 50) -> ()  [unwired: 1 out]
          }
        }
        n528 = VISA Clear(VISA resource name=w1267, error in (no error)=w1268) -> (VISA resource name out=w1263:refnum<visa-resource-name>, error out=w1266:errorcluster)
        n529 = local write "VISA resource name out"(w1263) -> ()
      }
      event "BK3": Value Change {
        n530 = event-data() -> ("NewVal"=w1302:bool)  [unwired: 1 in]
        n531 = flat-sequence {
          tunnel: w1302 -> [w1307]
          tunnel: refnum<visa-resource-name> "Adam" ("VISA resource name") -> [w1306]
          tunnel: w1300 -> [w1305]
          tunnel: [w1304] -> w1296
          tunnel: [w1303] -> w1295
          tunnel: [w1323] -> w1298
          tunnel: [w1324] -> w1299
          tunnel: w1296 -> [w1324]
          tunnel: w1295 -> [w1323]
          frame #0 {
            n532 = case shown="True" w1307 {
              tunnel: [w1309 w1318] -> w1304
              tunnel: [w1308 w1317] -> w1303
              tunnel: w1305 -> [w1311 w1316]
              tunnel: w1306 -> [w1310 w1315]
              frame False {
                n533 = Concatenate Strings("#051400" ("string"), "\r\n") -> (w1314:string)
                n534 = VISA Write(VISA resource name=w1310, write buffer=w1314, error in (no error)=w1311) -> (VISA resource name out=w1308:refnum<visa-resource-name>, error out=w1309:errorcluster)  [unwired: 1 out]
              }
              frame True {
                n535 = Concatenate Strings("#051401" ("string"), "\r\n") -> (w1321:string)
                n536 = VISA Write(VISA resource name=w1315, write buffer=w1321, error in (no error)=w1316) -> (VISA resource name out=w1317:refnum<visa-resource-name>, error out=w1318:errorcluster)  [unwired: 1 out]
              }
            }
          }
          frame #1 {
            n537 = Wait (ms)(milliseconds to wait=u32 50) -> ()  [unwired: 1 out]
          }
        }
        n538 = VISA Clear(VISA resource name=w1298, error in (no error)=w1299) -> (VISA resource name out=w1294:refnum<visa-resource-name>, error out=w1297:errorcluster)
        n539 = local write "VISA resource name out"(w1294) -> ()
      }
      event "F-R VISAR 4": Value Change {
        n540 = event-data() -> ("NewVal"=w1333:bool)  [unwired: 1 in]
        n541 = flat-sequence {
          tunnel: w1333 -> [w1338]
          tunnel: refnum<visa-resource-name> "Adam" ("VISA resource name") -> [w1337]
          tunnel: w1331 -> [w1336]
          tunnel: [w1335] -> w1327
          tunnel: [w1334] -> w1326
          tunnel: [w1354] -> w1329
          tunnel: [w1355] -> w1330
          tunnel: w1327 -> [w1355]
          tunnel: w1326 -> [w1354]
          frame #0 {
            n542 = case shown="True" w1338 {
              tunnel: [w1342 w1349] -> w1335
              tunnel: [w1341 w1348] -> w1334
              tunnel: w1337 -> [w1340 w1346]
              tunnel: w1336 -> [w1339 w1347]
              frame False {
                n543 = Concatenate Strings("#051500" ("string"), "\r\n") -> (w1345:string)
                n544 = VISA Write(VISA resource name=w1340, write buffer=w1345, error in (no error)=w1339) -> (VISA resource name out=w1341:refnum<visa-resource-name>, error out=w1342:errorcluster)  [unwired: 1 out]
              }
              frame True {
                n545 = Concatenate Strings("#051501" ("string"), "\r\n") -> (w1352:string)
                n546 = VISA Write(VISA resource name=w1346, write buffer=w1352, error in (no error)=w1347) -> (VISA resource name out=w1348:refnum<visa-resource-name>, error out=w1349:errorcluster)  [unwired: 1 out]
              }
            }
          }
          frame #1 {
            n547 = Wait (ms)(milliseconds to wait=u32 50) -> ()  [unwired: 1 out]
          }
        }
        n548 = VISA Clear(VISA resource name=w1329, error in (no error)=w1330) -> (VISA resource name out=w1325:refnum<visa-resource-name>, error out=w1328:errorcluster)
        n549 = local write "VISA resource name out"(w1325) -> ()
      }
      event "F-R VISAR 3": Value Change {
        n550 = event-data() -> ("NewVal"=w1364:bool)  [unwired: 1 in]
        n551 = flat-sequence {
          tunnel: w1364 -> [w1369]
          tunnel: refnum<visa-resource-name> "Adam" ("VISA resource name") -> [w1368]
          tunnel: w1362 -> [w1367]
          tunnel: [w1366] -> w1358
          tunnel: [w1365] -> w1357
          tunnel: [w1385] -> w1360
          tunnel: [w1386] -> w1361
          tunnel: w1358 -> [w1386]
          tunnel: w1357 -> [w1385]
          frame #0 {
            n552 = case shown="True" w1369 {
              tunnel: [w1373 w1379] -> w1366
              tunnel: [w1372 w1380] -> w1365
              tunnel: w1367 -> [w1371 w1378]
              tunnel: w1368 -> [w1370 w1377]
              frame False {
                n553 = Concatenate Strings("#051600" ("string"), "\r\n") -> (w1376:string)
                n554 = VISA Write(VISA resource name=w1370, write buffer=w1376, error in (no error)=w1371) -> (VISA resource name out=w1372:refnum<visa-resource-name>, error out=w1373:errorcluster)  [unwired: 1 out]
              }
              frame True {
                n555 = Concatenate Strings("#051601" ("string"), "\r\n") -> (w1383:string)
                n556 = VISA Write(VISA resource name=w1377, write buffer=w1383, error in (no error)=w1378) -> (VISA resource name out=w1380:refnum<visa-resource-name>, error out=w1379:errorcluster)  [unwired: 1 out]
              }
            }
          }
          frame #1 {
            n557 = Wait (ms)(milliseconds to wait=u32 50) -> ()  [unwired: 1 out]
          }
        }
        n558 = VISA Clear(VISA resource name=w1360, error in (no error)=w1361) -> (VISA resource name out=w1356:refnum<visa-resource-name>, error out=w1359:errorcluster)
        n559 = local write "VISA resource name out"(w1356) -> ()
      }
      event "FI": Value Change {
        n560 = event-data() -> ("NewVal"=w1395:bool)  [unwired: 1 in]
        n561 = flat-sequence {
          tunnel: w1395 -> [w1400]
          tunnel: w1394 -> [w1399]
          tunnel: refnum<visa-resource-name> "Adam" ("VISA resource name") -> [w1398]
          tunnel: [w1397] -> w1389
          tunnel: [w1396] -> w1388
          tunnel: [w1416] -> w1391
          tunnel: [w1417] -> w1392
          tunnel: w1389 -> [w1417]
          tunnel: w1388 -> [w1416]
          frame #0 {
            n562 = case shown="True" w1400 {
              tunnel: w1399 -> [w1404 w1408]
              tunnel: w1398 -> [w1403 w1409]
              tunnel: [w1402 w1411] -> w1397
              tunnel: [w1401 w1410] -> w1396
              frame False {
                n563 = Concatenate Strings("#051700" ("string"), "\r\n") -> (w1407:string)
                n564 = VISA Write(VISA resource name=w1403, write buffer=w1407, error in (no error)=w1404) -> (VISA resource name out=w1401:refnum<visa-resource-name>, error out=w1402:errorcluster)  [unwired: 1 out]
              }
              frame True {
                n565 = Concatenate Strings("#051701" ("string"), "\r\n") -> (w1414:string)
                n566 = VISA Write(VISA resource name=w1409, write buffer=w1414, error in (no error)=w1408) -> (VISA resource name out=w1410:refnum<visa-resource-name>, error out=w1411:errorcluster)  [unwired: 1 out]
              }
            }
          }
          frame #1 {
            n567 = Wait (ms)(milliseconds to wait=u32 50) -> ()  [unwired: 1 out]
          }
        }
        n568 = VISA Clear(VISA resource name=w1391, error in (no error)=w1392) -> (VISA resource name out=w1387:refnum<visa-resource-name>, error out=w1390:errorcluster)
        n569 = local write "VISA resource name out"(w1387) -> ()
      }
      event "rele 0_6": Value Change {
        n570 = event-data() -> ("NewVal"=w1426:bool)  [unwired: 1 in]
        n571 = flat-sequence {
          tunnel: w1426 -> [w1431]
          tunnel: refnum<visa-resource-name> "Adam" ("VISA resource name") -> [w1430]
          tunnel: w1424 -> [w1429]
          tunnel: [w1428] -> w1420
          tunnel: [w1427] -> w1419
          tunnel: [w1447] -> w1422
          tunnel: [w1448] -> w1423
          tunnel: w1420 -> [w1448]
          tunnel: w1419 -> [w1447]
          frame #0 {
            n572 = case shown="True" w1431 {
              tunnel: [w1435 w1442] -> w1427
              tunnel: [w1434 w1441] -> w1428
              tunnel: w1429 -> [w1433 w1440]
              tunnel: w1430 -> [w1432 w1439]
              frame False {
                n573 = Concatenate Strings("#061000" ("string"), "\r\n") -> (w1438:string)
                n574 = VISA Write(VISA resource name=w1432, write buffer=w1438, error in (no error)=w1433) -> (VISA resource name out=w1435:refnum<visa-resource-name>, error out=w1434:errorcluster)  [unwired: 1 out]
              }
              frame True {
                n575 = Concatenate Strings("#061001" ("string"), "\r\n") -> (w1445:string)
                n576 = VISA Write(VISA resource name=w1439, write buffer=w1445, error in (no error)=w1440) -> (VISA resource name out=w1442:refnum<visa-resource-name>, error out=w1441:errorcluster)  [unwired: 1 out]
              }
            }
          }
          frame #1 {
            n577 = Wait (ms)(milliseconds to wait=u32 50) -> ()  [unwired: 1 out]
          }
        }
        n578 = VISA Clear(VISA resource name=w1422, error in (no error)=w1423) -> (VISA resource name out=w1418:refnum<visa-resource-name>, error out=w1421:errorcluster)
        n579 = local write "VISA resource name out"(w1418) -> ()
      }
      event "F0-ethernet 4": Value Change {
        n580 = event-data() -> ("NewVal"=w1457:bool)  [unwired: 1 in]
        n581 = flat-sequence {
          tunnel: w1457 -> [w1462]
          tunnel: refnum<visa-resource-name> "Adam" ("VISA resource name") -> [w1461]
          tunnel: w1455 -> [w1460]
          tunnel: [w1459] -> w1451
          tunnel: [w1458] -> w1450
          tunnel: [w1478] -> w1453
          tunnel: [w1479] -> w1454
          tunnel: w1451 -> [w1479]
          tunnel: w1450 -> [w1478]
          frame #0 {
            n582 = case shown="True" w1462 {
              tunnel: [w1466 w1473] -> w1459
              tunnel: [w1465 w1472] -> w1458
              tunnel: w1460 -> [w1464 w1471]
              tunnel: w1461 -> [w1463 w1470]
              frame False {
                n583 = Concatenate Strings("#061100" ("string"), "\r\n") -> (w1469:string)
                n584 = VISA Write(VISA resource name=w1463, write buffer=w1469, error in (no error)=w1464) -> (VISA resource name out=w1465:refnum<visa-resource-name>, error out=w1466:errorcluster)  [unwired: 1 out]
              }
              frame True {
                n585 = Concatenate Strings("#061101" ("string"), "\r\n") -> (w1476:string)
                n586 = VISA Write(VISA resource name=w1470, write buffer=w1476, error in (no error)=w1471) -> (VISA resource name out=w1472:refnum<visa-resource-name>, error out=w1473:errorcluster)  [unwired: 1 out]
              }
            }
          }
          frame #1 {
            n587 = Wait (ms)(milliseconds to wait=u32 50) -> ()  [unwired: 1 out]
          }
        }
        n588 = VISA Clear(VISA resource name=w1453, error in (no error)=w1454) -> (VISA resource name out=w1449:refnum<visa-resource-name>, error out=w1452:errorcluster)
        n589 = local write "VISA resource name out"(w1449) -> ()
      }
      event "F0-ethernet 5": Value Change {
        n590 = event-data() -> ("NewVal"=w1488:bool)  [unwired: 1 in]
        n591 = flat-sequence {
          tunnel: w1488 -> [w1493]
          tunnel: refnum<visa-resource-name> "Adam" ("VISA resource name") -> [w1492]
          tunnel: w1486 -> [w1491]
          tunnel: [w1490] -> w1482
          tunnel: [w1489] -> w1481
          tunnel: [w1509] -> w1484
          tunnel: [w1510] -> w1485
          tunnel: w1482 -> [w1510]
          tunnel: w1481 -> [w1509]
          frame #0 {
            n592 = case shown="True" w1493 {
              tunnel: [w1495 w1504] -> w1490
              tunnel: [w1494 w1503] -> w1489
              tunnel: w1492 -> [w1497 w1502]
              tunnel: w1491 -> [w1496 w1501]
              frame False {
                n593 = Concatenate Strings("#061200" ("string"), "\r\n") -> (w1500:string)
                n594 = VISA Write(VISA resource name=w1497, write buffer=w1500, error in (no error)=w1496) -> (VISA resource name out=w1494:refnum<visa-resource-name>, error out=w1495:errorcluster)  [unwired: 1 out]
              }
              frame True {
                n595 = Concatenate Strings("#061201" ("string"), "\r\n") -> (w1507:string)
                n596 = VISA Write(VISA resource name=w1502, write buffer=w1507, error in (no error)=w1501) -> (VISA resource name out=w1503:refnum<visa-resource-name>, error out=w1504:errorcluster)  [unwired: 1 out]
              }
            }
          }
          frame #1 {
            n597 = Wait (ms)(milliseconds to wait=u32 50) -> ()  [unwired: 1 out]
          }
        }
        n598 = VISA Clear(VISA resource name=w1484, error in (no error)=w1485) -> (VISA resource name out=w1480:refnum<visa-resource-name>, error out=w1483:errorcluster)
        n599 = local write "VISA resource name out"(w1480) -> ()
      }
      event "F0-ethernet 1": Value Change {
        n600 = event-data() -> ("NewVal"=w1519:bool)  [unwired: 1 in]
        n601 = flat-sequence {
          tunnel: w1519 -> [w1524]
          tunnel: refnum<visa-resource-name> "Adam" ("VISA resource name") -> [w1523]
          tunnel: w1517 -> [w1522]
          tunnel: [w1521] -> w1513
          tunnel: [w1520] -> w1512
          tunnel: [w1540] -> w1515
          tunnel: [w1541] -> w1516
          tunnel: w1513 -> [w1541]
          tunnel: w1512 -> [w1540]
          frame #0 {
            n602 = case shown="True" w1524 {
              tunnel: w1523 -> [w1528 w1535]
              tunnel: w1522 -> [w1527 w1534]
              tunnel: [w1526 w1532] -> w1521
              tunnel: [w1525 w1533] -> w1520
              frame False {
                n603 = Concatenate Strings("#061300" ("string"), "\r\n") -> (w1531:string)
                n604 = VISA Write(VISA resource name=w1528, write buffer=w1531, error in (no error)=w1527) -> (VISA resource name out=w1525:refnum<visa-resource-name>, error out=w1526:errorcluster)  [unwired: 1 out]
              }
              frame True {
                n605 = Concatenate Strings("#061301" ("string"), "\r\n") -> (w1538:string)
                n606 = VISA Write(VISA resource name=w1535, write buffer=w1538, error in (no error)=w1534) -> (VISA resource name out=w1533:refnum<visa-resource-name>, error out=w1532:errorcluster)  [unwired: 1 out]
              }
            }
          }
          frame #1 {
            n607 = Wait (ms)(milliseconds to wait=u32 50) -> ()  [unwired: 1 out]
          }
        }
        n608 = VISA Clear(VISA resource name=w1515, error in (no error)=w1516) -> (VISA resource name out=w1511:refnum<visa-resource-name>, error out=w1514:errorcluster)
        n609 = local write "VISA resource name out"(w1511) -> ()
      }
      event "F0-ethernet 2": Value Change {
        n610 = event-data() -> ("NewVal"=w1550:bool)  [unwired: 1 in]
        n611 = flat-sequence {
          tunnel: w1550 -> [w1555]
          tunnel: refnum<visa-resource-name> "Adam" ("VISA resource name") -> [w1554]
          tunnel: w1548 -> [w1553]
          tunnel: [w1552] -> w1544
          tunnel: [w1551] -> w1543
          tunnel: [w1571] -> w1546
          tunnel: [w1572] -> w1547
          tunnel: w1544 -> [w1572]
          tunnel: w1543 -> [w1571]
          frame #0 {
            n612 = case shown="True" w1555 {
              tunnel: [w1557 w1566] -> w1552
              tunnel: [w1556 w1565] -> w1551
              tunnel: w1553 -> [w1559 w1564]
              tunnel: w1554 -> [w1558 w1563]
              frame False {
                n613 = Concatenate Strings("#061400" ("string"), "\r\n") -> (w1562:string)
                n614 = VISA Write(VISA resource name=w1558, write buffer=w1562, error in (no error)=w1559) -> (VISA resource name out=w1556:refnum<visa-resource-name>, error out=w1557:errorcluster)  [unwired: 1 out]
              }
              frame True {
                n615 = Concatenate Strings("#061401" ("string"), "\r\n") -> (w1569:string)
                n616 = VISA Write(VISA resource name=w1563, write buffer=w1569, error in (no error)=w1564) -> (VISA resource name out=w1565:refnum<visa-resource-name>, error out=w1566:errorcluster)  [unwired: 1 out]
              }
            }
          }
          frame #1 {
            n617 = Wait (ms)(milliseconds to wait=u32 50) -> ()  [unwired: 1 out]
          }
        }
        n618 = VISA Clear(VISA resource name=w1546, error in (no error)=w1547) -> (VISA resource name out=w1542:refnum<visa-resource-name>, error out=w1545:errorcluster)
        n619 = local write "VISA resource name out"(w1542) -> ()
      }
      event "PZS 1 DOP": Value Change {
        n620 = event-data() -> ("NewVal"=w1581:bool)  [unwired: 1 in]
        n621 = flat-sequence {
          tunnel: w1581 -> [w1586]
          tunnel: refnum<visa-resource-name> "Adam" ("VISA resource name") -> [w1585]
          tunnel: w1579 -> [w1584]
          tunnel: [w1583] -> w1575
          tunnel: [w1582] -> w1574
          tunnel: [w1602] -> w1577
          tunnel: [w1603] -> w1578
          tunnel: w1575 -> [w1603]
          tunnel: w1574 -> [w1602]
          frame #0 {
            n622 = case shown="True" w1586 {
              tunnel: [w1590 w1597] -> w1583
              tunnel: [w1589 w1596] -> w1582
              tunnel: w1585 -> [w1588 w1594]
              tunnel: w1584 -> [w1587 w1595]
              frame False {
                n623 = Concatenate Strings("#061500" ("string"), "\r\n") -> (w1593:string)
                n624 = VISA Write(VISA resource name=w1588, write buffer=w1593, error in (no error)=w1587) -> (VISA resource name out=w1589:refnum<visa-resource-name>, error out=w1590:errorcluster)  [unwired: 1 out]
              }
              frame True {
                n625 = Concatenate Strings("#061501" ("string"), "\r\n") -> (w1600:string)
                n626 = VISA Write(VISA resource name=w1594, write buffer=w1600, error in (no error)=w1595) -> (VISA resource name out=w1596:refnum<visa-resource-name>, error out=w1597:errorcluster)  [unwired: 1 out]
              }
            }
          }
          frame #1 {
            n627 = Wait (ms)(milliseconds to wait=u32 50) -> ()  [unwired: 1 out]
          }
        }
        n628 = VISA Clear(VISA resource name=w1577, error in (no error)=w1578) -> (VISA resource name out=w1573:refnum<visa-resource-name>, error out=w1576:errorcluster)
        n629 = local write "VISA resource name out"(w1573) -> ()
      }
      event "PZS 2 DOP": Value Change {
        n630 = event-data() -> ("NewVal"=w1612:bool)  [unwired: 1 in]
        n631 = flat-sequence {
          tunnel: w1612 -> [w1617]
          tunnel: refnum<visa-resource-name> "Adam" ("VISA resource name") -> [w1616]
          tunnel: w1610 -> [w1615]
          tunnel: [w1614] -> w1606
          tunnel: [w1613] -> w1605
          tunnel: [w1633] -> w1608
          tunnel: [w1634] -> w1609
          tunnel: w1606 -> [w1634]
          tunnel: w1605 -> [w1633]
          frame #0 {
            n632 = case shown="True" w1617 {
              tunnel: [w1621 w1627] -> w1614
              tunnel: [w1620 w1628] -> w1613
              tunnel: w1615 -> [w1619 w1626]
              tunnel: w1616 -> [w1618 w1625]
              frame False {
                n633 = Concatenate Strings("#061600" ("string"), "\r\n") -> (w1624:string)
                n634 = VISA Write(VISA resource name=w1618, write buffer=w1624, error in (no error)=w1619) -> (VISA resource name out=w1620:refnum<visa-resource-name>, error out=w1621:errorcluster)  [unwired: 1 out]
              }
              frame True {
                n635 = Concatenate Strings("#061601" ("string"), "\r\n") -> (w1631:string)
                n636 = VISA Write(VISA resource name=w1625, write buffer=w1631, error in (no error)=w1626) -> (VISA resource name out=w1628:refnum<visa-resource-name>, error out=w1627:errorcluster)  [unwired: 1 out]
              }
            }
          }
          frame #1 {
            n637 = Wait (ms)(milliseconds to wait=u32 50) -> ()  [unwired: 1 out]
          }
        }
        n638 = VISA Clear(VISA resource name=w1608, error in (no error)=w1609) -> (VISA resource name out=w1604:refnum<visa-resource-name>, error out=w1607:errorcluster)
        n639 = local write "VISA resource name out"(w1604) -> ()
      }
      event "F0-ethernet 3": Value Change {
        n640 = event-data() -> ("NewVal"=w1643:bool)  [unwired: 1 in]
        n641 = flat-sequence {
          tunnel: w1643 -> [w1648]
          tunnel: refnum<visa-resource-name> "Adam" ("VISA resource name") -> [w1647]
          tunnel: w1641 -> [w1646]
          tunnel: [w1645] -> w1637
          tunnel: [w1644] -> w1636
          tunnel: [w1664] -> w1639
          tunnel: [w1665] -> w1640
          tunnel: w1637 -> [w1665]
          tunnel: w1636 -> [w1664]
          frame #0 {
            n642 = case shown="True" w1648 {
              tunnel: w1646 -> [w1652 w1656]
              tunnel: w1647 -> [w1651 w1657]
              tunnel: [w1650 w1659] -> w1645
              tunnel: [w1649 w1658] -> w1644
              frame False {
                n643 = Concatenate Strings("#061700" ("string"), "\r\n") -> (w1655:string)
                n644 = VISA Write(VISA resource name=w1651, write buffer=w1655, error in (no error)=w1652) -> (VISA resource name out=w1649:refnum<visa-resource-name>, error out=w1650:errorcluster)  [unwired: 1 out]
              }
              frame True {
                n645 = Concatenate Strings("#061701" ("string"), "\r\n") -> (w1662:string)
                n646 = VISA Write(VISA resource name=w1657, write buffer=w1662, error in (no error)=w1656) -> (VISA resource name out=w1658:refnum<visa-resource-name>, error out=w1659:errorcluster)  [unwired: 1 out]
              }
            }
          }
          frame #1 {
            n647 = Wait (ms)(milliseconds to wait=u32 50) -> ()  [unwired: 1 out]
          }
        }
        n648 = VISA Clear(VISA resource name=w1639, error in (no error)=w1640) -> (VISA resource name out=w1635:refnum<visa-resource-name>, error out=w1638:errorcluster)
        n649 = local write "VISA resource name out"(w1635) -> ()
      }
    }
    "error out" <- w7
    "error out 2" <- w6
    n650 = Get Date/Time In Seconds() -> (seconds since 1Jan1904=→"Time Stamp":timestamp)
    n651 = VISA Close(VISA resource name=w12, error in (no error)=w7) -> (error out=w13:errorcluster)
    n652 = VISA Close(VISA resource name=w11, error in (no error)=w10) -> ()  [unwired: 1 out]
    n653 = VISA Close(VISA resource name=w8, error in (no error)=w9) -> ()  [unwired: 1 out]
  }
